vi "Periodic Tasks.vi"(8 "error in":errorcluster) -> (0 "error out":errorcluster)   [LabVIEW 2018]
doc: "This VI runs in parallel to other tasks. It can contain as many user-defined periodic loops as you need. These can carry out PID or other sorts of timed response."
uses:
  <vilib>/Rock Robotics/WPI/Joystick/WPI_JoystickDevRef.ctl
  <vilib>/Rock Robotics/WPI/Joystick/WPI_JoystickDeviceEnum.ctl
  <vilib>/Rock Robotics/WPI/RobotDrive/WPI_RobotDriveDevRef.ctl
  <vilib>/Rock Robotics/WPI/MotorControl/WPI_MotorControlDeviceRef.ctl
  <vilib>/Rock Robotics/WPI/MotorControl/WPI_MotorControlType.ctl
  <vilib>/Rock Robotics/SystemInterfaces/DIO/FPGA_DIOPWMChannel.ctl
  <vilib>/Rock Robotics/WPI/PWM/WPI_PWMDeadband.ctl
  <vilib>/Rock Robotics/SystemInterfaces/DIO/FPGA_DIOChannel.ctl
  <vilib>/Rock Robotics/WPI/Solenoid/WPI_SolenoidDevRef.ctl
  <vilib>/Rock Robotics/WPI/Solenoid/WPI_SolenoidChannel.ctl
  <vilib>/Rock Robotics/WPI/DigitalInput/WPI_DigitalInputDevRef.ctl
  Vision States.ctl
  <vilib>/Rock Robotics/WPI/DriverStation/WPI_DriverStationRobotMode2.ctl
  Hatch Retainer States.ctl
  HAB Bk Spd Motor States.ctl
  Hatch Kicking States.ctl
  <vilib>/Rock Robotics/WPI/Solenoid/WPI_SolenoidValue.ctl
  <vilib>/Rock Robotics/WPI/ThirdParty/Phoenix-LabVIEW/Motor Controller/Controls/CTRE_Phoenix_MotorControl_ControlMode.ctl
  <vilib>/Rock Robotics/WPI/ThirdParty/Phoenix-LabVIEW/Motor Controller/Controls/CTRE_Phoenix_MotorControl_MotionProfileTrajectoryPoint.ctl
  <vilib>/Rock Robotics/WPI/Utilities/WPI_GetSetVariantRefNum.vi
  <vilib>/Rock Robotics/WPI/ThirdParty/Phoenix-LabVIEW/Motor Controller/Get/CTRE_Phoenix_MotorController_GetQuadratureData.vi
  Robot Global Data.vi
  <vilib>/Rock Robotics/Network Tables/NT Write Boolean.vi
  <vilib>/Rock Robotics/WPI/Solenoid/WPI_SolenoidSetEnum.vi
  <vilib>/addons/control/pid/pid.llb/PID (DBL).vi
  <vilib>/Rock Robotics/Network Tables/NT Write Number.vi
  <vilib>/Rock Robotics/WPI/ThirdParty/Phoenix-LabVIEW/Motor Controller/Closed Loop/Motion Profile/CTRE_Phoenix_MotorControl_BufferedTrajectoryPointStream_WriteAll.vi
  <vilib>/Rock Robotics/Network Tables/NT Read Number.vi
  <vilib>/addons/control/pid/NI_PID_pid.lvlib
panel:
  in  "FRDriveMotorDevRef":T1={"DeviceStatus"={"status"=FALSE, "code"=0, "source"=""}, "Type"=enum."PWM", "PWM"={"PWM Channel"=enum."Invalid", "DeadBand"={"Name"="", "maxPositivePwm"=0, "minPositivePwm"=0, "centerPwm"=0, "maxNegativePwm"=0, "minNegativePwm"=0, "angularRange"=0}}, "CAN"={"Device Number"=0, "SetOutput VI Ref"=variant(refnum<vi> refnum), "GetOutput VI Ref"=variant(refnum<vi> refnum), "Enable VI Ref"=variant(refnum<vi> refnum), "Disable VI Ref"=variant(refnum<vi> refnum), "Data"=variant}, "Invert"=FALSE, "DIO PWM"={"PWM \"Enable\" Channel"=enum."Invalid", "DIOChannel"=enum."Invalid", "PWM Rate"=0.0}}
  in  "FLDriveMotorDevRef":T1={"DeviceStatus"={"status"=FALSE, "code"=0, "source"=""}, "Type"=enum."PWM", "PWM"={"PWM Channel"=enum."Invalid", "DeadBand"={"Name"="", "maxPositivePwm"=0, "minPositivePwm"=0, "centerPwm"=0, "maxNegativePwm"=0, "minNegativePwm"=0, "angularRange"=0}}, "CAN"={"Device Number"=0, "SetOutput VI Ref"=variant(refnum<vi> refnum), "GetOutput VI Ref"=variant(refnum<vi> refnum), "Enable VI Ref"=variant(refnum<vi> refnum), "Disable VI Ref"=variant(refnum<vi> refnum), "Data"=variant}, "Invert"=FALSE, "DIO PWM"={"PWM \"Enable\" Channel"=enum."Invalid", "DIOChannel"=enum."Invalid", "PWM Rate"=0.0}}
  in  "HAB3DriveModuleMotorDevRef 2":T1={"DeviceStatus"={"status"=FALSE, "code"=0, "source"=""}, "Type"=enum."PWM", "PWM"={"PWM Channel"=enum."Invalid", "DeadBand"={"Name"="", "maxPositivePwm"=0, "minPositivePwm"=0, "centerPwm"=0, "maxNegativePwm"=0, "minNegativePwm"=0, "angularRange"=0}}, "CAN"={"Device Number"=0, "SetOutput VI Ref"=variant(refnum<vi> refnum), "GetOutput VI Ref"=variant(refnum<vi> refnum), "Enable VI Ref"=variant(refnum<vi> refnum), "Disable VI Ref"=variant(refnum<vi> refnum), "Data"=variant}, "Invert"=FALSE, "DIO PWM"={"PWM \"Enable\" Channel"=enum."Invalid", "DIOChannel"=enum."Invalid", "PWM Rate"=0.0}}
  in  "BkSpdAdjusterMotorDevRef":T1={"DeviceStatus"={"status"=FALSE, "code"=0, "source"=""}, "Type"=enum."PWM", "PWM"={"PWM Channel"=enum."Invalid", "DeadBand"={"Name"="", "maxPositivePwm"=0, "minPositivePwm"=0, "centerPwm"=0, "maxNegativePwm"=0, "minNegativePwm"=0, "angularRange"=0}}, "CAN"={"Device Number"=0, "SetOutput VI Ref"=variant(refnum<vi> refnum), "GetOutput VI Ref"=variant(refnum<vi> refnum), "Enable VI Ref"=variant(refnum<vi> refnum), "Disable VI Ref"=variant(refnum<vi> refnum), "Data"=variant}, "Invert"=FALSE, "DIO PWM"={"PWM \"Enable\" Channel"=enum."Invalid", "DIOChannel"=enum."Invalid", "PWM Rate"=0.0}}
  in  "HABAssisterSolenoidDevRef":T6={"DevStatus"={"status"=FALSE, "code"=0, "source"=""}, "Pneumatics Control Module"=0, "Forward Solenoid Channel"=enum."Invalid", "Reverse Solenoid Channel"=enum."Invalid"}
  out "Right Traj. Pts Array":dbl[][](array[numeric])
  out "Left Traj. Pts Array":dbl[][](array[numeric])
  in  "Back HAB 3 Limit Switch":T8={"DevStatus"={"status"=FALSE, "code"=0, "source"=""}, "DIO Channel"=enum."Invalid"}
  in  "Front HAB 3 Limit Switch":T8={"DevStatus"={"status"=FALSE, "code"=0, "source"=""}, "DIO Channel"=enum."Invalid"}
  in  "BottomRetainerSwitchDevRef":T8={"DevStatus"={"status"=FALSE, "code"=0, "source"=""}, "DIO Channel"=enum."Invalid"}
  in  "TopRetainerSwitchDevRef":T8={"DevStatus"={"status"=FALSE, "code"=0, "source"=""}, "DIO Channel"=enum."Invalid"}
  in  "HatchRetainerMotorDevRef":T1={"DeviceStatus"={"status"=FALSE, "code"=0, "source"=""}, "Type"=enum."PWM", "PWM"={"PWM Channel"=enum."Invalid", "DeadBand"={"Name"="", "maxPositivePwm"=0, "minPositivePwm"=0, "centerPwm"=0, "maxNegativePwm"=0, "minNegativePwm"=0, "angularRange"=0}}, "CAN"={"Device Number"=0, "SetOutput VI Ref"=variant(refnum<vi> refnum), "GetOutput VI Ref"=variant(refnum<vi> refnum), "Enable VI Ref"=variant(refnum<vi> refnum), "Disable VI Ref"=variant(refnum<vi> refnum), "Data"=variant}, "Invert"=FALSE, "DIO PWM"={"PWM \"Enable\" Channel"=enum."Invalid", "DIOChannel"=enum."Invalid", "PWM Rate"=0.0}}
  in  "HAB3BackSolenoidDevRef":T6={"DevStatus"={"status"=FALSE, "code"=0, "source"=""}, "Pneumatics Control Module"=0, "Forward Solenoid Channel"=enum."Invalid", "Reverse Solenoid Channel"=enum."Invalid"}
  in  "HAB3FrontSolenoidDevRef":T6={"DevStatus"={"status"=FALSE, "code"=0, "source"=""}, "Pneumatics Control Module"=0, "Forward Solenoid Channel"=enum."Invalid", "Reverse Solenoid Channel"=enum."Invalid"}
  in  "AuxJoystickDevRef":T9={"Device"=enum."USB 1"}
  in  "DriveJoystickDevRef":T9={"Device"=enum."USB 1"}
  in  "HAB3DriveModuleMotorDevRef":T1={"DeviceStatus"={"status"=FALSE, "code"=0, "source"=""}, "Type"=enum."PWM", "PWM"={"PWM Channel"=enum."Invalid", "DeadBand"={"Name"="", "maxPositivePwm"=0, "minPositivePwm"=0, "centerPwm"=0, "maxNegativePwm"=0, "minNegativePwm"=0, "angularRange"=0}}, "CAN"={"Device Number"=0, "SetOutput VI Ref"=variant(refnum<vi> refnum), "GetOutput VI Ref"=variant(refnum<vi> refnum), "Enable VI Ref"=variant(refnum<vi> refnum), "Disable VI Ref"=variant(refnum<vi> refnum), "Data"=variant}, "Invert"=FALSE, "DIO PWM"={"PWM \"Enable\" Channel"=enum."Invalid", "DIOChannel"=enum."Invalid", "PWM Rate"=0.0}}
  in  "LifterSolenoidDevRef":T6={"DevStatus"={"status"=FALSE, "code"=0, "source"=""}, "Pneumatics Control Module"=0, "Forward Solenoid Channel"=enum."Invalid", "Reverse Solenoid Channel"=enum."Invalid"}
  in  "DriveJoystickDevRef":T9={"Device"=enum."USB 1"}
  in  "HatchCollectorMotorDevRef":T1={"DeviceStatus"={"status"=FALSE, "code"=0, "source"=""}, "Type"=enum."PWM", "PWM"={"PWM Channel"=enum."Invalid", "DeadBand"={"Name"="", "maxPositivePwm"=0, "minPositivePwm"=0, "centerPwm"=0, "maxNegativePwm"=0, "minNegativePwm"=0, "angularRange"=0}}, "CAN"={"Device Number"=0, "SetOutput VI Ref"=variant(refnum<vi> refnum), "GetOutput VI Ref"=variant(refnum<vi> refnum), "Enable VI Ref"=variant(refnum<vi> refnum), "Disable VI Ref"=variant(refnum<vi> refnum), "Data"=variant}, "Invert"=FALSE, "DIO PWM"={"PWM \"Enable\" Channel"=enum."Invalid", "DIOChannel"=enum."Invalid", "PWM Rate"=0.0}}
  in  "AuxJoystickDevRef":T9
  in  "RetainerSolenoidDevRef":T6={"DevStatus"={"status"=FALSE, "code"=0, "source"=""}, "Pneumatics Control Module"=0, "Forward Solenoid Channel"=enum."Invalid", "Reverse Solenoid Channel"=enum."Invalid"}
  in  "KickerSolenoidDevRef":T6={"DevStatus"={"status"=FALSE, "code"=0, "source"=""}, "Pneumatics Control Module"=0, "Forward Solenoid Channel"=enum."Invalid", "Reverse Solenoid Channel"=enum."Invalid"}
  in  "Drive Motors":T11={"DevStatus"={"status"=FALSE, "code"=0, "source"=""}, "Motors[]"=[], "Square Inputs"=FALSE, "Max Output"=1.0}
  in  "AuxJoystickDevRef":T9={"Device"=enum."USB 1"}
  in  "DriveJoystickDevRef":T9
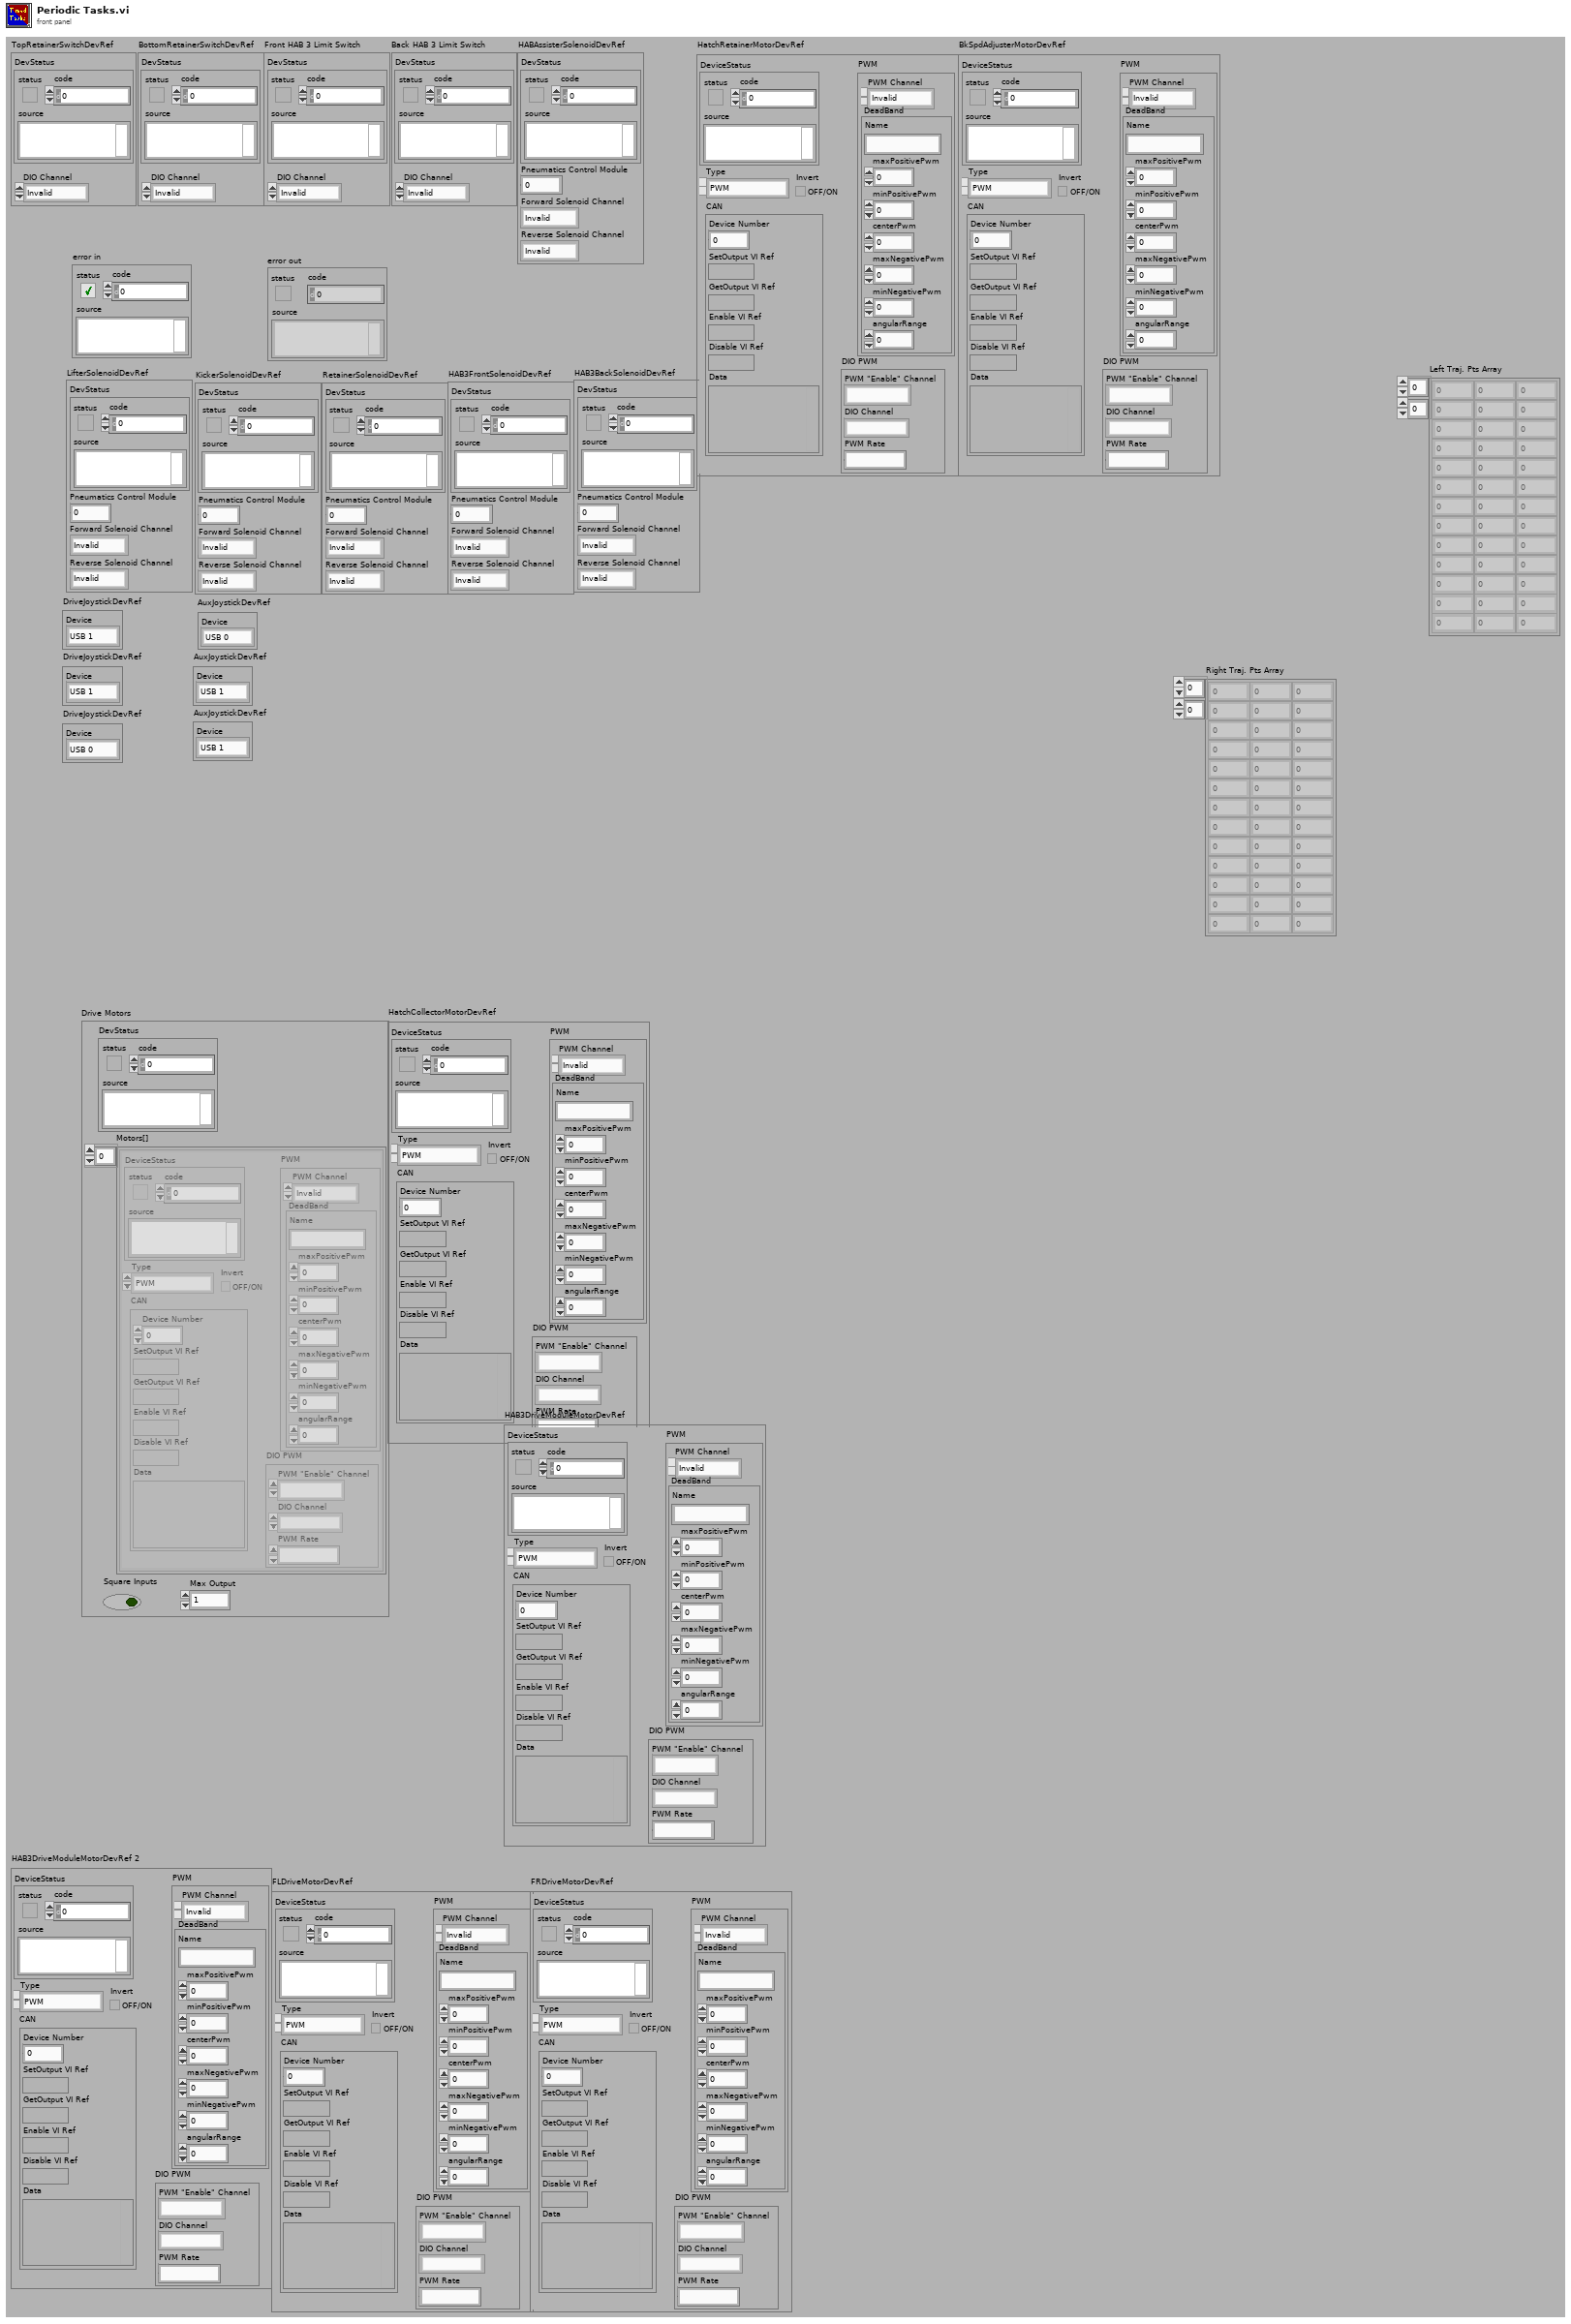
[diagram p1: front panel]
types:
  T1 = typedef "WPI_MotorControlDeviceRef.ctl" = cluster{"DeviceStatus":errorcluster, "Type":T2, "PWM":cluster{"PWM Channel":T3, "DeadBand":T4}, "CAN":cluster{"Device Number":u8, "SetOutput VI Ref":variant, "GetOutput VI Ref":variant, "Enable VI Ref":variant, "Disable VI Ref":variant, "Data":variant}, "Invert":bool, "DIO PWM":cluster{"PWM \"Enable\" Channel":T3, "DIOChannel":T5, "PWM Rate":dbl}}
  T2 = typedef "WPI_MotorControlType.ctl" = enum16{"PWM", "CAN", "DIO PWM"}
  T3 = typedef "FPGA_DIOPWMChannel.ctl" = enum8{"PWM 0", "PWM 1", "PWM 2", "PWM 3", "PWM 4", "PWM 5", "PWM 6", "PWM 7", "PWM 8", "PWM 9", "PWM MXP 0", "PWM MXP 1", "PWM MXP 2", "PWM MXP 3", "PWM MXP 4", "PWM MXP 5", "PWM MXP 6", "PWM MXP 7", "PWM MXP 8", "PWM MXP 9", "Invalid"}
  T4 = typedef "WPI_PWMDeadband.ctl" = cluster{"Name":string, "maxPositivePwm":i32, "minPositivePwm":i32, "centerPwm":i32, "maxNegativePwm":i32, "minNegativePwm":i32, "angularRange":u16}
  T5 = typedef "FPGA_DIOChannel.ctl" = enum8{"DIO 0", "DIO 1", "DIO 2", "DIO 3", "DIO 4", "DIO 5", "DIO 6", "DIO 7", "DIO 8", "DIO 9", "DIO MXP 0", "DIO MXP 1", "DIO MXP 2", "DIO MXP 3", "DIO MXP 4", "DIO MXP 5", "DIO MXP 6", "DIO MXP 7", "DIO MXP 8", "DIO MXP 9", "DIO MXP 10", "DIO MXP 11", "DIO MXP 12", "DIO MXP 13", "DIO MXP 14", "DIO MXP 15", "SPI Port CS1", "SPI Port CS2", "SPI Port CS3", "SPI Port MISO", "SPI Port MOSI", "Invalid"}
  T6 = typedef "WPI_SolenoidDevRef.ctl" = cluster{"DevStatus":errorcluster, "Pneumatics Control Module":u8, "Forward Solenoid Channel":T7, "Reverse Solenoid Channel":T7}
  T7 = typedef "WPI_SolenoidChannel.ctl" = enum8{"Solenoid 0", "Solenoid 1", "Solenoid 2", "Solenoid 3", "Solenoid 4", "Solenoid 5", "Solenoid 6", "Solenoid 7", "Invalid"}
  T8 = typedef "WPI_DigitalInputDevRef.ctl" = cluster{"DevStatus":errorcluster, "DIO Channel":T5}
  T9 = typedef "WPI_JoystickDevRef.ctl" = cluster{"Device":T10}
  T10 = typedef "WPI_JoystickDeviceEnum.ctl" = enum16{"USB 0", "USB 1", "USB 2", "USB 3", "USB 4", "USB 5"}
  T11 = typedef "WPI_RobotDriveDevRef.ctl" = cluster{"DevStatus":errorcluster, "Motors[]":T1[], "Square Inputs":bool, "Max Output":dbl}
  T12 = typedef "Hatch Kicking States.ctl" = enum16{"Ready", "Stop Retaining Hatch", "Kick Hatch"}
  T13 = typedef "HAB Bk Spd Motor States.ctl" = enum16{"Fully Up", "Going Down", "Fully Down", "Going Up"}
  T14 = typedef "Hatch Retainer States.ctl" = enum16{"Fully Down (not retained)", "Going Up", "Fully Up (retained)", "Going Down"}
  T15 = cluster{"X Button":i32, "A Button":i32, "B Button":i32, "Y Button":i32, "LB Button":i32, "RB Button":i32, "LT Button":i32, "RT Button":i32, "BACK Button":i32, "START Button":i32, "LJ Click Button":i32, "RJ Click Button":i32}
  T16 = cluster{"Left X":i32, "Left Y":i32, "Right X":i32, "Right Y":i32}
  T17 = typedef "WPI_DriverStationRobotMode2.ctl" = enum16{"Autonomous Disabled", "Autonomous Enabled", "Teleop Disabled", "Teleop Enabled", "Disconnected", "Finish", "Test Disabled", "Test Enabled", "Emergency Stopped"}
  T18 = cluster{"offsetAngle H":dbl, "offsetAngle V":dbl, "area":dbl, "skew":dbl, "shortest side (pxls)":dbl, "longest side (pxls)":dbl}
  T19 = typedef "Vision States.ctl" = enum16{"Ready", "Forward Until Target at Edge", "Vision Track"}
  T20 = cluster{"A Button":i32, "B Button":i32, "X Button":i32, "Y Button":i32, "LB Button":i32, "RB Button":i32, "BACK Button":i32, "START Button":i32, "LJ Click Button":i32, "RJ Click Button":i32}
  T21 = cluster{"Left X":i32, "Left Y":i32, "Right X":i32, "Right Y":i32, "RT Button":i32, "LT Button":i32}
  T22 = cluster{"MotorControlDevRef":T1, "MotorControlDevRef":T1}
  T23 = typedef "WPI_GyroDevRef.ctl" = cluster{"DevStatus":errorcluster, "Analog Channel":T24, "Gain (VoltsPerDegree/Second)":dbl, "Gyro Type":enum16{"Analog", "XRS450"}, "Handle":i32, "SPI Bus":T25, "Device Found":bool, "Sample Rate":dbl, "Calibrate On Open":bool, "Offset":dbl}
  T24 = typedef "FPGA_AIChannel.ctl" = enum8{"AI 0", "AI 1", "AI 2", "AI 3", "AI MXP 0", "AI MXP 1", "AI MXP 2", "AI MXP 3", "Invalid"}
  T25 = typedef "spi_bus.ctl" = enum16{"SPI On-Board, CS0", "SPI On-Board, CS1", "SPI On-Board, CS2", "SPI On-Board, CS3", "SPI MXP", "Invalid"}
  T26 = cluster{"Front Drive Motors":cluster{"FLDriveMotor":T1, "FRDriveMotor":T1}, "HAB3DriveModuleMotorDevRef 2":T1, "DriveJoystickDevRef":T9, "AuxJoystickDevRef":T9, "Drive Axes":dbl[], "Drive Buttons":bool[], "Drive POVs":i16[], "Aux Axes":dbl[], "Aux Buttons":bool[], "Aux POVs":i16[], "Robot Mode":T17, "Drive Motors":T11, "Drive Axes Indexes":cluster{"Left X":i32, "Left Y":i32, "Right X":i32, "Right Y":i32, "RT Button":i32, "LT Button":i32}, "Drive Button Indexes":cluster{"A Button":i32, "B Button":i32, "X Button":i32, "Y Button":i32, "LB Button":i32, "RB Button":i32, "BACK Button":i32, "START Button":i32, "LJ Click Button":i32, "RJ Click Button":i32}, "Joystick VS Vision Latch":bool, "Vision States":T19, "limelight":cluster{"offsetAngle H":dbl, "offsetAngle V":dbl, "area":dbl, "skew":dbl, "shortest side (pxls)":dbl, "longest side (pxls)":dbl}, "Vision Track Mode Override":bool, "T = Motion Profile, F = Percent Output":bool, "Arcade Drive?":bool, "Start Motion Profile?":bool}
  T27 = cluster{"TopRetainerSwitchDevRef":T8, "BottomRetainerSwitchDevRef":T8, "HatchRetainerMotorDevRef":T1, "LifterSolenoidDevRef":T6, "DriveJoystickDevRef":T9, "KickerSolenoidDevRef":T6, "RetainerSolenoidDevRef":T6, "AuxJoystickDevRef":T9, "HatchCollectorMotorDevRef":T1, "Drive Axes":dbl[], "Drive Buttons":bool[], "Drive POVs":i16[], "Aux Axes":dbl[], "Aux Buttons":bool[], "Aux POVs":i16[], "Robot Mode":T17, "Aux Joystick Indexes":cluster{"Left X":i32, "Left Y":i32, "Right X":i32, "Right Y":i32}, "Aux Button Indexes":cluster{"X Button":i32, "A Button":i32, "B Button":i32, "Y Button":i32, "LB Button":i32, "RB Button":i32, "LT Button":i32, "RT Button":i32, "BACK Button":i32, "START Button":i32, "LJ Click Button":i32, "RJ Click Button":i32}, "Hatch Retainer Move Up/Down":bool, "Hatch Collector Actual Angle":dbl, "Hatch Collector Wanted Angle":dbl, "Hatch Retainer States":T14, "Hatch Kicking States":T12}
  T28 = cluster{"BkSpdAdjusterMotorDevRef":T1, "HABAssisterSolenoidDevRef":T6, "Back HAB 3 Limit Switch":T8, "Front HAB 3 Limit Switch":T8, "HAB3DriveModuleMotorDevRef":T1, "DriveJoystickDevRef":T9, "AuxJoystickDevRef":T9, "HAB3FrontSolenoidDevRef":T6, "HAB3BackSolenoidDevRef":T6, "Drive Axes":dbl[], "Drive Buttons":bool[], "Drive POVs":i16[], "Aux Axes":dbl[], "Aux Buttons":bool[], "Aux POVs":i16[], "Robot Mode":T17, "Aux Joystick Indexes":cluster{"Left X":i32, "Left Y":i32, "Right X":i32, "Right Y":i32}, "Aux Button Indexes":cluster{"X Button":i32, "A Button":i32, "B Button":i32, "Y Button":i32, "LB Button":i32, "RB Button":i32, "LT Button":i32, "RT Button":i32, "BACK Button":i32, "START Button":i32, "LJ Click Button":i32, "RJ Click Button":i32}, "Front Cylinders Latch":bool, "Back Cylinders Latch":bool, "Yaw":dbl, "Pitch":dbl, "Roll":dbl, "HAB Bk Spd Motor States":T13}
  T29 = typedef "CTRE_Phoenix_MotorControl_MotionProfileTrajectoryPoint.ctl" = cluster{"Position":dbl, "Velocity":dbl, "Arbitrary Feed Forward":dbl, "Auxiliary Position":dbl, "Auxiliary Velocity":dbl, "Auxiliary Arbitrary Feed Forward":dbl, "Profile Slot Select":i32, "Auxiliary Profile Slot Select":i32, "isLastPoint?":bool, "Zero Position?":bool, "durationMs":u32, "Use Aux PID?":bool}
  T30 = typedef "Which Robot Enum.ctl" = enum16{"Competition Bot", "Practice Bot", "Code Bot"}
  T31 = typedef "CTRE_Phoenix_MotorControl_BufferedTrajectoryPointStream_DeviceRef.ctl" = cluster{"Handle":u64, "Library Path":path}
  T32 = typedef "WPI_SolenoidValue.ctl" = enum16{"Off", "On", "Forward", "Reverse"}
  T33 = cluster{"proportional gain (Kc)":dbl, "integral time (Ti, min)":dbl, "derivative time (Td, min)":dbl}
  T34 = typedef "CTRE_Phoenix_MotorControl_ControlMode.ctl" = u16
  T35 = cluster{"Yaw":dbl, "Roll":dbl, "Pitch":dbl, "Heading":dbl, "Fused Heading":dbl}
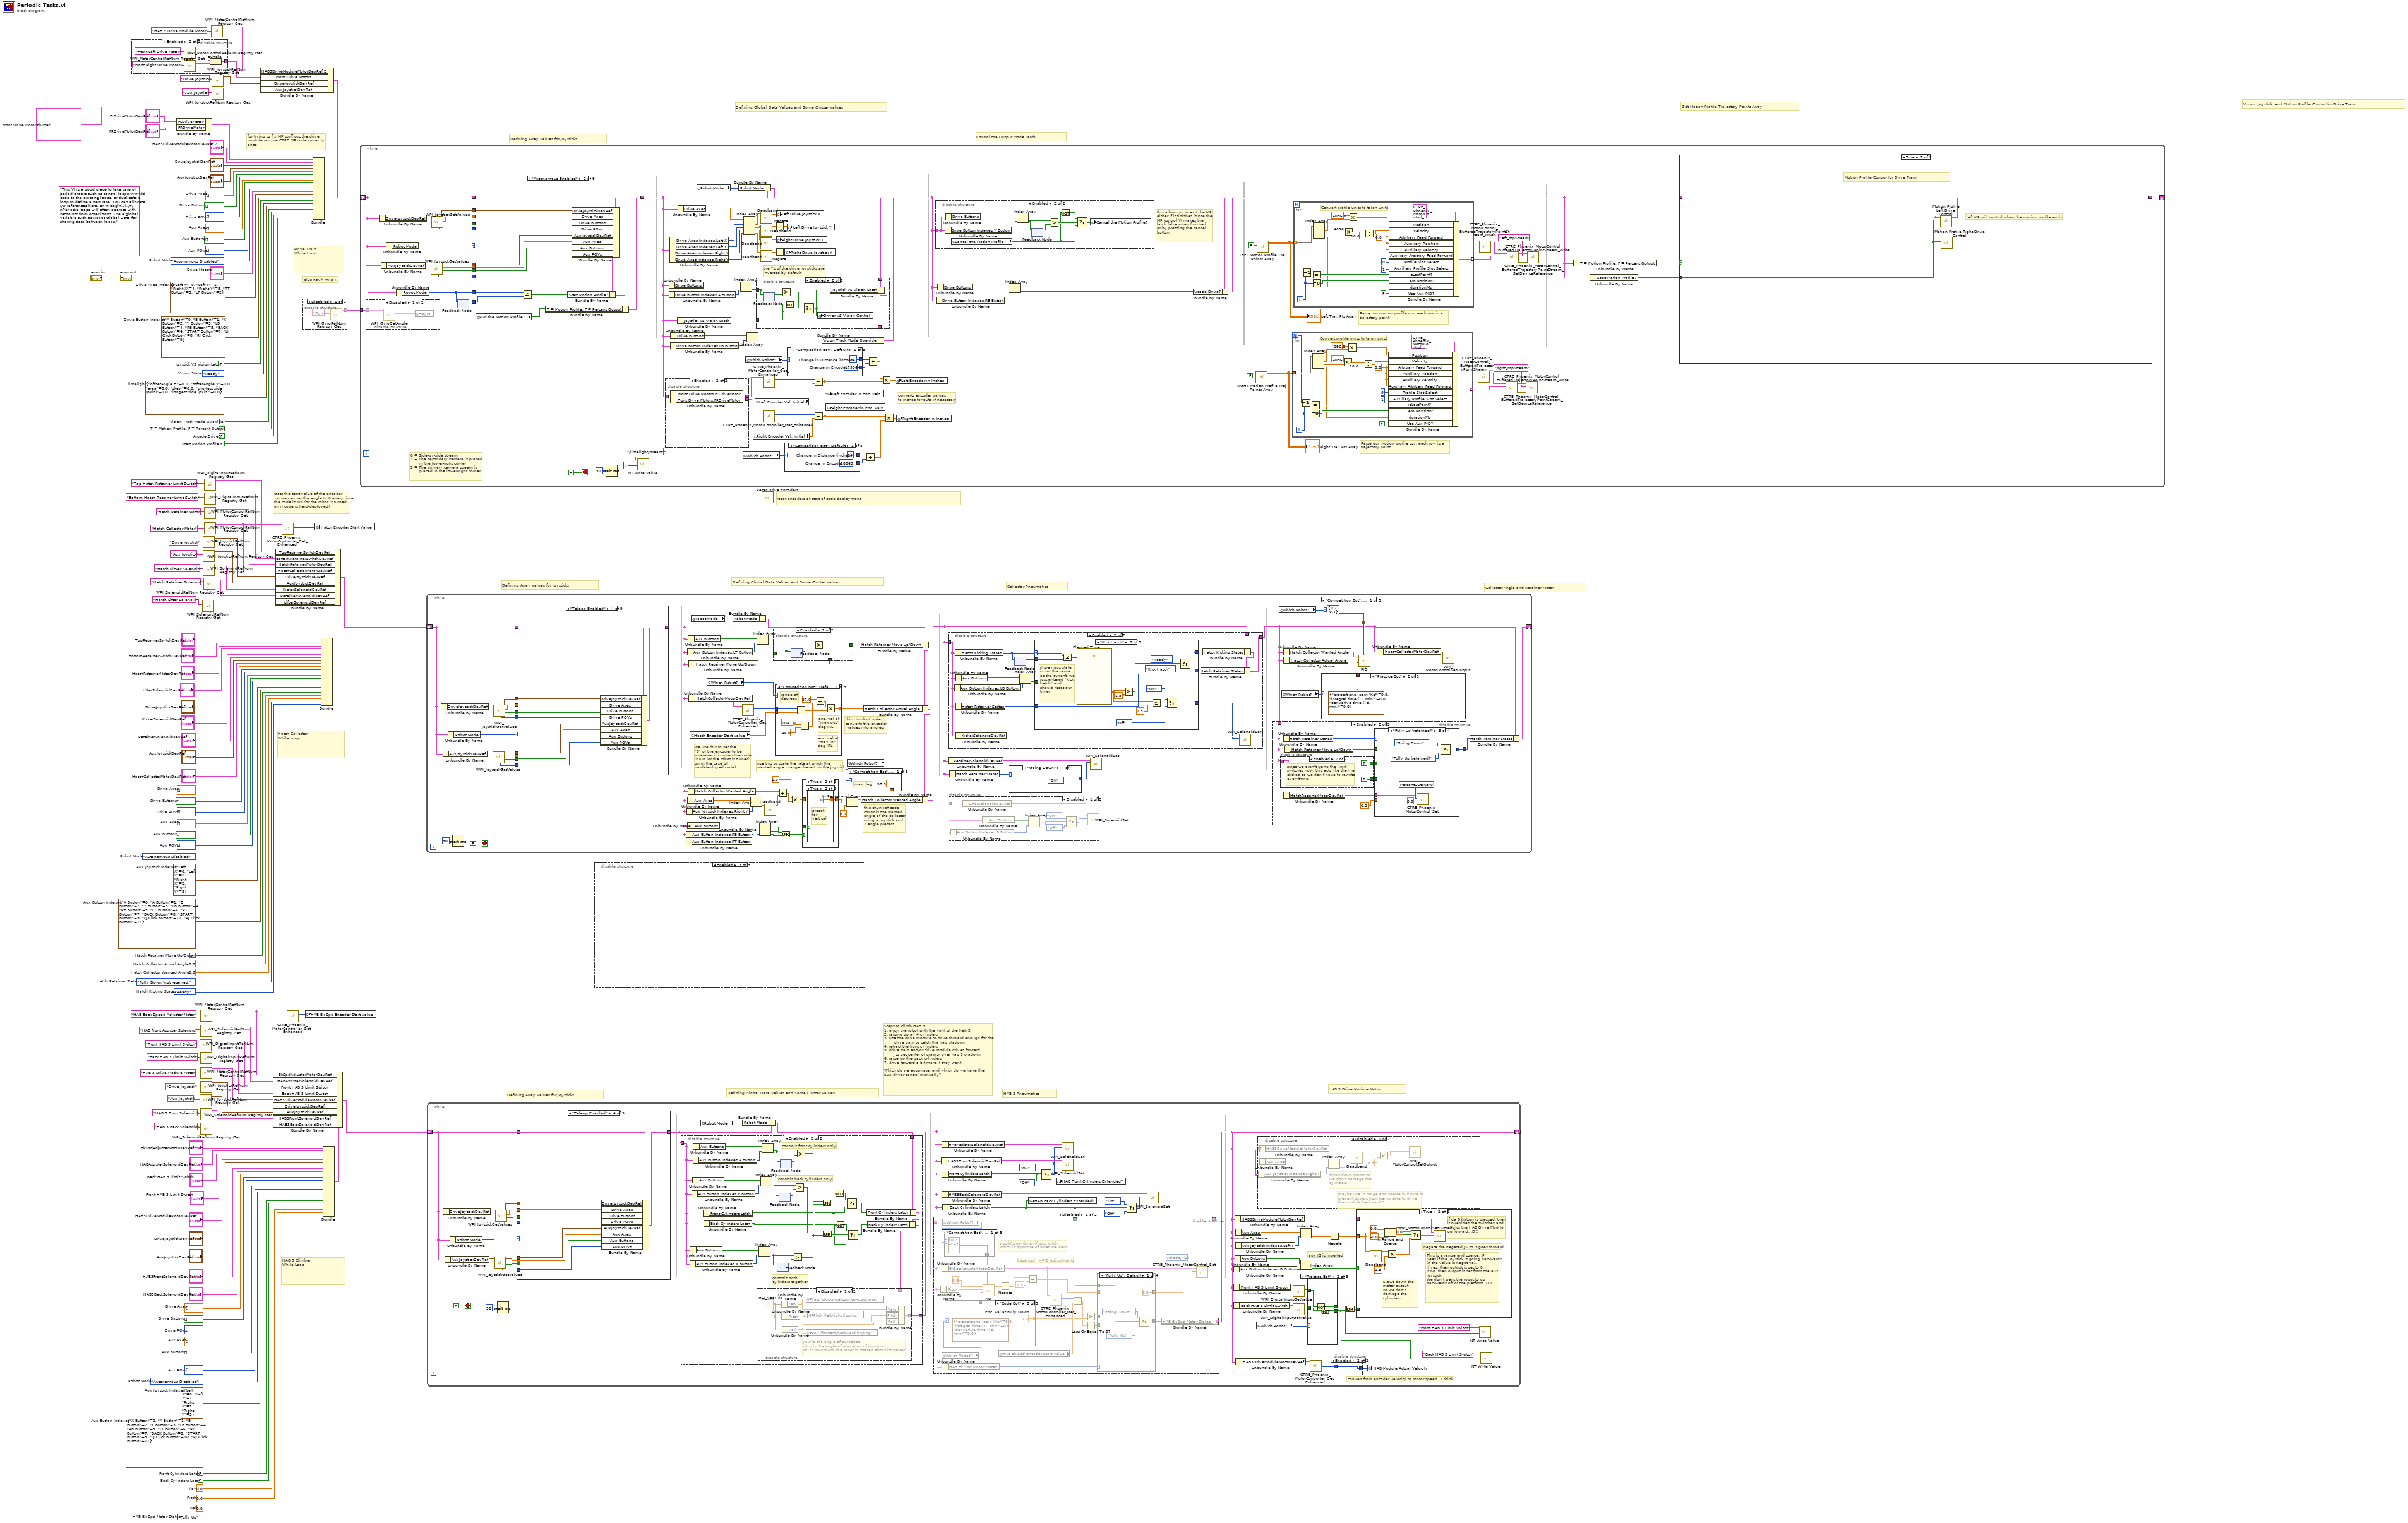
[diagram p0: block diagram]
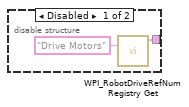
[diagram p2: hidden frame]
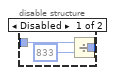
[diagram p3: hidden frame]
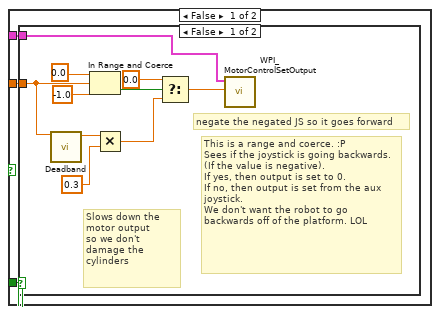
[diagram p4: hidden frame]
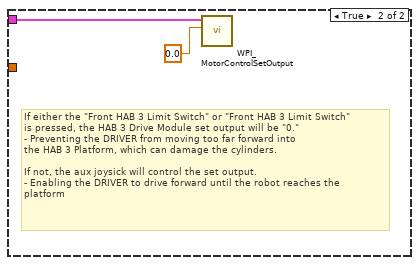
[diagram p5: hidden frame]
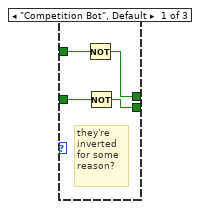
[diagram p6: hidden frame]
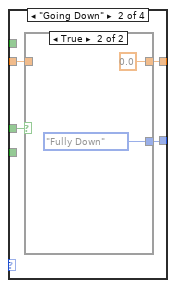
[diagram p8: hidden frame]
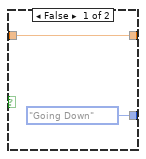
[diagram p9: hidden frame]
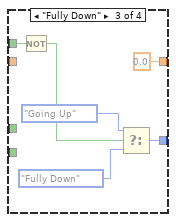
[diagram p10: hidden frame]
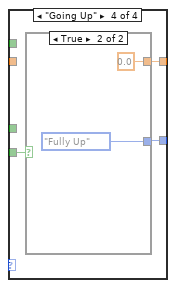
[diagram p11: hidden frame]
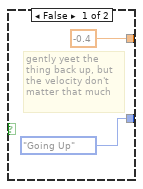
[diagram p12: hidden frame]
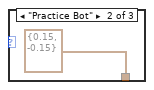
[diagram p13: hidden frame]
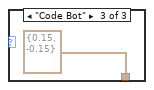
[diagram p14: hidden frame]
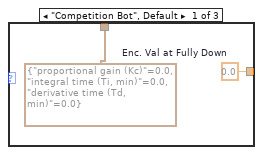
[diagram p15: hidden frame]
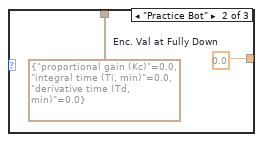
[diagram p16: hidden frame]
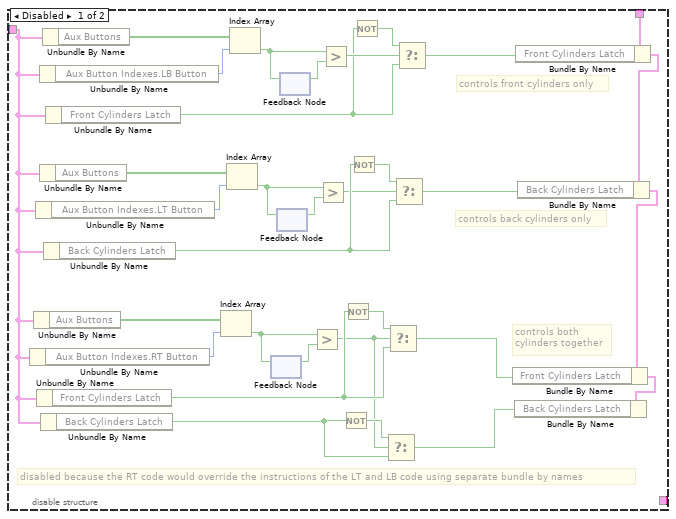
[diagram p18: hidden frame]
diagram:
  w1 = cluster{"FLDriveMotor":T1, "FRDriveMotor":T1} {"FLDriveMotor"={"DeviceStatus"={"status"=FALSE, "code"=0, "source"=""}, "Type"=enum."PWM", "PWM"={"PWM Channel"=enum."Invalid", "DeadBand"={"Name"="", "maxPositivePwm"=0, "minPositivePwm"=0, "centerPwm"=0, "maxNegativePwm"=0, "minNegativePwm"=0, "angularRange"=0}}, "CAN"={"Device Number"=0, "SetOutput VI Ref"=variant(refnum<vi> refnum), "GetOutput VI Ref"=variant(refnum<vi> refnum), "Enable VI Ref"=variant(refnum<vi> refnum), "Disable VI Ref"=variant(refnum<vi> refnum), "Data"=variant}, "Invert"=FALSE, "DIO PWM"={"PWM \"Enable\" Channel"=enum."Invalid", "DIOChannel"=enum."Invalid", "PWM Rate"=0.0}}, "FRDriveMotor"={"DeviceStatus"={"status"=FALSE, "code"=0, "source"=""}, "Type"=enum."PWM", "PWM"={"PWM Channel"=enum."Invalid", "DeadBand"={"Name"="", "maxPositivePwm"=0, "minPositivePwm"=0, "centerPwm"=0, "maxNegativePwm"=0, "minNegativePwm"=0, "angularRange"=0}}, "CAN"={"Device Number"=0, "SetOutput VI Ref"=variant(refnum<vi> refnum), "GetOutput VI Ref"=variant(refnum<vi> refnum), "Enable VI Ref"=variant(refnum<vi> refnum), "Disable VI Ref"=variant(refnum<vi> refnum), "Data"=variant}, "Invert"=FALSE, "DIO PWM"={"PWM \"Enable\" Channel"=enum."Invalid", "DIOChannel"=enum."Invalid", "PWM Rate"=0.0}}}  # Front Drive Motors
  w9 = FALSE  # Start Motion Profile?
  w10 = FALSE  # Arcade Drive?
  w11 = Hatch_Kicking_States."Ready"  # Hatch Kicking States
  w12 = HAB_Bk_Spd_Motor_States."Fully Up"  # HAB Bk Spd Motor States
  w17 = 0.0  # Roll
  w18 = 0.0  # Pitch
  w19 = 0.0  # Yaw
  w29 = Hatch_Retainer_States."Fully Down (not retained)"  # Hatch Retainer States
  w39 = FALSE  # T = Motion Profile, F = Percent Output
  w41 = 0.0  # Hatch Collector Wanted Angle
  w42 = FALSE  # Back Cylinders Latch
  w43 = FALSE  # Front Cylinders Latch
  w44 = T15 {"X Button"=0, "A Button"=1, "B Button"=2, "Y Button"=3, "LB Button"=4, "RB Button"=5, "LT Button"=6, "RT Button"=7, "BACK Button"=8, "START Button"=9, "LJ Click Button"=10, "RJ Click Button"=11}  # Aux Button Indexes
  w45 = T16 {"Left X"=0, "Left Y"=1, "Right X"=2, "Right Y"=3}  # Aux Joystick Indexes
  w46 = WPI_DriverStationRobotMode2."Autonomous Disabled"  # Robot Mode
  w47 = i16[] []  # Aux POVs
  w48 = bool[] []  # Aux Buttons
  w49 = dbl[] []  # Aux Axes
  w50 = i16[] []  # Drive POVs
  w51 = bool[] []  # Drive Buttons
  w52 = dbl[] []  # Drive Axes
  w75 = 0.0  # Hatch Collector Actual Angle
  w76 = FALSE  # Hatch Retainer Move Up/Down
  w77 = T15 {"X Button"=0, "A Button"=1, "B Button"=2, "Y Button"=3, "LB Button"=4, "RB Button"=5, "LT Button"=6, "RT Button"=7, "BACK Button"=8, "START Button"=9, "LJ Click Button"=10, "RJ Click Button"=11}  # Aux Button Indexes
  w78 = T16 {"Left X"=0, "Left Y"=1, "Right X"=2, "Right Y"=3}  # Aux Joystick Indexes
  w82 = WPI_DriverStationRobotMode2."Autonomous Disabled"  # Robot Mode
  w83 = i16[] []  # Aux POVs
  w84 = bool[] []  # Aux Buttons
  w85 = dbl[] []  # Aux Axes
  w86 = i16[] []  # Drive POVs
  w87 = bool[] []  # Drive Buttons
  w88 = dbl[] []  # Drive Axes
  w102 = FALSE  # Vision Track Mode Override
  w103 = T18 {"offsetAngle H"=0.0, "offsetAngle V"=0.0, "area"=0.0, "skew"=0.0, "shortest side (pxls)"=0.0, "longest side (pxls)"=0.0}  # limelight
  w104 = Vision_States."Ready"  # Vision States
  w105 = FALSE  # Joystick VS Vision Latch
  w106 = T20 {"A Button"=0, "B Button"=1, "X Button"=2, "Y Button"=3, "LB Button"=4, "RB Button"=5, "BACK Button"=6, "START Button"=7, "LJ Click Button"=8, "RJ Click Button"=9}  # Drive Button Indexes
  w108 = T21 {"Left X"=0, "Left Y"=1, "Right X"=4, "Right Y"=5, "RT Button"=3, "LT Button"=2}  # Drive Axes Indexes
  w112 = i16[] []  # Aux POVs
  w113 = bool[] []  # Aux Buttons
  w114 = dbl[] []  # Aux Axes
  w111 = WPI_DriverStationRobotMode2."Autonomous Disabled"  # Robot Mode
  w115 = i16[] []  # Drive POVs
  w116 = bool[] []  # Drive Buttons
  w117 = dbl[] []  # Drive Axes
  (unwired) "This VI is a good place to take care of periodic tasks such as control loops.\n\nAdd code to the existing loops, or duplicate a loop to define a new rate. You can allocate I/O references here, or in Begin.vi.\n\nPeriodic loops will often operate with setpoints from other loops. Use a global variable such as Robot Global Data for sharing data between loops."
  # "HAB 3 Drive Module Motor"
  # "HAB 3 Pneumatics"
  # "Steps to climb HAB 3\n1. align the robot with the front of the hab 3\n2. raising up all 4 cylinders\n3. use the drive module to drive forward enough for the \n        drive train to catch the hab platform\n4. retract the front cylinders\n5. drive train and/or drive module drives forward \n         to get center of gravity over hab 3 platform\n6. raise up the back cylinders\n7. drive forward a bit more if they want\n\nWhich do we automate, and which do we have the \naux driver control manually?"
  # "Defining Global Data Values and Some Cluster Values"
  # "Defining Array Values for Joysticks"
  # "Collector Angle and Retainer Motor"
  # "Collector Pneumatics"
  # "Defining Global Data Values and Some Cluster Values"
  # "Defining Array Values for Joysticks"
  # "for trying to fix MP stuff cuz the drive\nmodule ran the CTRE MP code correctly\nonce"
  # "reset encoders at start of code deployment"
  # "Get Motion Profile Trajectory Points Array"
  # "Control the Output Mode Latch"
  # "plus navX mxp :-)"
  # "Gets the start value of the encoder\n so we can set the angle to 0 every time\nthe code is run (or the robot is turned\non if code is hard-deployed)"
  # "HAB 3 Climber\nWhile Loop"
  # "Hatch Collector\nWhile Loop"
  # "Drive Train\nWhile Loop"
  # "Vision, Joystick, and Motion Profile Control for Drive Train"
  # "Defining Array Values for Joysticks"
  # "Defining Global Data Values and Some Cluster Values"
  n1 = disable-structure shown="Enabled" {
    disable-tunnel: [w126 w129] -> w109
    frame Disabled {
      n2 = call <vilib>:"WPI_RobotDriveRefNum Registry Get.vi"("refnum name"="Drive Motors") -> ("RobotDriveDevRef"=w126:T11)  [unwired: 9 in, 1 out]
    }
    frame Enabled {
      n3 = call <vilib>:"WPI_MotorControlRefNum Registry Get.vi"("refnum name"="Front Left Drive Motor") -> ("MotorControlDevRef"=w130:T1)  [unwired: 9 in, 1 out]
      n4 = call <vilib>:"WPI_MotorControlRefNum Registry Get.vi"("refnum name"="Front Right Drive Motor") -> ("MotorControlDevRef"=w131:T1)  [unwired: 9 in, 1 out]
      n5 = Bundle("MotorControlDevRef"=w130, "MotorControlDevRef"=w131) -> (w129:T22)  [unwired: 1 in]
    }
  }
  n6 = Bundle By Name(cluster=w1, "FLDriveMotor"="FLDriveMotorDevRef", "FRDriveMotor"="FRDriveMotorDevRef") -> (w2:cluster{"FLDriveMotor":T1, "FRDriveMotor":T1})
  n7 = call <vilib>:"WPI_DigitalInputRefNum Registry Get.vi"("refnum name"="Front HAB 3 Limit Switch") -> ("DigitalInputDevRef"=w24:T8)  [unwired: 9 in, 1 out]
  n8 = call <vilib>:"WPI_JoystickRefNum Registry Get.vi"("refnum name"="Aux Joystick") -> ("JoystickDevRef"=w56:T9)  [unwired: 9 in, 1 out]
  n9 = call <vilib>:"WPI_SolenoidRefNum Registry Get.vi"("refnum name"="HAB Front Assister Solenoid") -> ("SolenoidDevRef"=w20:T6)  [unwired: 9 in, 1 out]
  n10 = call <vilib>:"WPI_DigitalInputRefNum Registry Get.vi"("refnum name"="Back HAB 3 Limit Switch") -> ("DigitalInputDevRef"=w23:T8)  [unwired: 9 in, 1 out]
  n11 = call <vilib>:"WPI_MotorControlRefNum Registry Get.vi"("refnum name"="HAB 3 Drive Module Motor") -> ("MotorControlDevRef"=w54:T1)  [unwired: 9 in, 1 out]
  n12 = call <vilib>:"WPI_JoystickRefNum Registry Get.vi"("refnum name"="Drive Joystick") -> ("JoystickDevRef"=w55:T9)  [unwired: 9 in, 1 out]
  n13 = call <vilib>:"WPI_SolenoidRefNum Registry Get.vi"("refnum name"="HAB 3 Front Solenoid") -> ("SolenoidDevRef"=w57:T6)  [unwired: 9 in, 1 out]
  n14 = call <vilib>:"WPI_MotorControlRefNum Registry Get.vi"("refnum name"="HAB Back Speed Adjuster Motor") -> ("MotorControlDevRef"=w13:T1)  [unwired: 9 in, 1 out]
  n15 = call <vilib>:"WPI_SolenoidRefNum Registry Get.vi"("refnum name"="HAB 3 Back Solenoid") -> ("SolenoidDevRef"=w58:T6)  [unwired: 9 in, 1 out]
  n16 = call <vilib>:"WPI_SolenoidRefNum Registry Get.vi"("refnum name"="Hatch Lifter Solenoid") -> ("SolenoidDevRef"=w71:T6)  [unwired: 9 in, 1 out]
  n17 = call <vilib>:"WPI_JoystickRefNum Registry Get.vi"("refnum name"="Aux Joystick") -> ("JoystickDevRef"=w93:T9)  [unwired: 9 in, 1 out]
  n18 = call <vilib>:"WPI_JoystickRefNum Registry Get.vi"("refnum name"="Drive Joystick") -> ("JoystickDevRef"=w79:T9)  [unwired: 9 in, 1 out]
  n19 = call <vilib>:"WPI_SolenoidRefNum Registry Get.vi"("refnum name"="Hatch Kicker Solenoid") -> ("SolenoidDevRef"=w96:T6)  [unwired: 9 in, 1 out]
  n20 = call <vilib>:"WPI_SolenoidRefNum Registry Get.vi"("refnum name"="Hatch Retainer Solenoid") -> ("SolenoidDevRef"=w95:T6)  [unwired: 9 in, 1 out]
  n21 = call <vilib>:"WPI_DigitalInputRefNum Registry Get.vi"("refnum name"="Top Hatch Retainer Limit Switch") -> ("DigitalInputDevRef"=w30:T8)  [unwired: 9 in, 1 out]
  n22 = call <vilib>:"WPI_DigitalInputRefNum Registry Get.vi"("refnum name"="Bottom Hatch Retainer Limit Switch") -> ("DigitalInputDevRef"=w31:T8)  [unwired: 9 in, 1 out]
  n23 = call <vilib>:"WPI_MotorControlRefNum Registry Get.vi"("refnum name"="Hatch Retainer Motor") -> ("MotorControlDevRef"=w36:T1)  [unwired: 9 in, 1 out]
  n24 = call <vilib>:"WPI_MotorControlRefNum Registry Get.vi"("refnum name"="Hatch Collector Motor") -> ("MotorControlDevRef"=w74:T1)  [unwired: 9 in, 1 out]
  n25 = call <vilib>:"WPI_MotorControlRefNum Registry Get.vi"("refnum name"="HAB 3 Drive Module Motor") -> ("MotorControlDevRef"=w6:T1)  [unwired: 9 in, 1 out]
  n26 = call <vilib>:"WPI_JoystickRefNum Registry Get.vi"("refnum name"="Drive Joystick") -> ("JoystickDevRef"=w120:T9)  [unwired: 9 in, 1 out]
  n27 = call <vilib>:"WPI_JoystickRefNum Registry Get.vi"("refnum name"="Aux Joystick") -> ("JoystickDevRef"=w119:T9)  [unwired: 9 in, 1 out]
  n28 = call-poly <vilib>:"CTRE_Phoenix_MotorController_Get_Enhanced.vi"("PhoenixMotorControlDevRef"=w74) -> ("Quadrature Position"=w73:i32)  [unwired: 11 in, 3 out]
  n29 = call-poly <vilib>:"CTRE_Phoenix_MotorController_Get_Enhanced.vi"("PhoenixMotorControlDevRef"=w13) -> ("Quadrature Position"=w14:i32)  [unwired: 11 in, 3 out]
  n30 = disable-structure shown="Disabled" {
    disable-tunnel: [w132 _] -> w40
    frame Disabled {
      n31 = call <vilib>:"WPI_GyroRefNum Registry Get.vi"("refnum name"="Gyro") -> ("GyroDevRef"=w132:T23)  [unwired: 9 in, 1 out]
    }
    frame Enabled {
    }
  }
  n32 = global write "Robot Global Data.vi" "HAB Bk Spd Encoder Start Value"(w14) -> ()
  n33 = Bundle("Front Drive Motors"=w2, "HAB3DriveModuleMotorDevRef 2"="HAB3DriveModuleMotorDevRef 2", "DriveJoystickDevRef"="DriveJoystickDevRef", "AuxJoystickDevRef"="AuxJoystickDevRef", "Drive Axes"=w117, "Drive Buttons"=w116, "Drive POVs"=w115, "Aux Axes"=w114, "Aux Buttons"=w113, "Aux POVs"=w112, "Robot Mode"=w111, "Drive Motors"="Drive Motors", "Drive Axes Indexes"=w108, "Drive Button Indexes"=w106, "Joystick VS Vision Latch"=w105, "Vision States"=w104, "limelight"=w103, "Vision Track Mode Override"=w102, "T = Motion Profile, F = Percent Output"=w39, "Arcade Drive?"=w10, "Start Motion Profile?"=w9) -> (w121:T26)  [unwired: 1 in]
  n34 = Bundle By Name(cluster=w121, "HAB3DriveModuleMotorDevRef 2"=w6, "Front Drive Motors"=w109, "DriveJoystickDevRef"=w120, "AuxJoystickDevRef"=w119) -> (w118:T26)
  n35 = global write "Robot Global Data.vi" "Hatch Encoder Start Value"(w73) -> ()
  n36 = Bundle("TopRetainerSwitchDevRef"="TopRetainerSwitchDevRef", "BottomRetainerSwitchDevRef"="BottomRetainerSwitchDevRef", "HatchRetainerMotorDevRef"="HatchRetainerMotorDevRef", "LifterSolenoidDevRef"="LifterSolenoidDevRef", "DriveJoystickDevRef"="DriveJoystickDevRef", "KickerSolenoidDevRef"="KickerSolenoidDevRef", "RetainerSolenoidDevRef"="RetainerSolenoidDevRef", "AuxJoystickDevRef"="AuxJoystickDevRef", "HatchCollectorMotorDevRef"="HatchCollectorMotorDevRef", "Drive Axes"=w88, "Drive Buttons"=w87, "Drive POVs"=w86, "Aux Axes"=w85, "Aux Buttons"=w84, "Aux POVs"=w83, "Robot Mode"=w82, "Aux Joystick Indexes"=w78, "Aux Button Indexes"=w77, "Hatch Retainer Move Up/Down"=w76, "Hatch Collector Actual Angle"=w75, "Hatch Collector Wanted Angle"=w41, "Hatch Retainer States"=w29, "Hatch Kicking States"=w11) -> (w99:T27)  [unwired: 1 in]
  n37 = Bundle By Name(cluster=w99, "TopRetainerSwitchDevRef"=w30, "BottomRetainerSwitchDevRef"=w31, "HatchRetainerMotorDevRef"=w36, "HatchCollectorMotorDevRef"=w74, "DriveJoystickDevRef"=w79, "AuxJoystickDevRef"=w93, "KickerSolenoidDevRef"=w96, "RetainerSolenoidDevRef"=w95, "LifterSolenoidDevRef"=w71) -> (w89:T27)
  n38 = Bundle("BkSpdAdjusterMotorDevRef"="BkSpdAdjusterMotorDevRef", "HABAssisterSolenoidDevRef"="HABAssisterSolenoidDevRef", "Back HAB 3 Limit Switch"="Back HAB 3 Limit Switch", "Front HAB 3 Limit Switch"="Front HAB 3 Limit Switch", "HAB3DriveModuleMotorDevRef"="HAB3DriveModuleMotorDevRef", "DriveJoystickDevRef"="DriveJoystickDevRef", "AuxJoystickDevRef"="AuxJoystickDevRef", "HAB3FrontSolenoidDevRef"="HAB3FrontSolenoidDevRef", "HAB3BackSolenoidDevRef"="HAB3BackSolenoidDevRef", "Drive Axes"=w52, "Drive Buttons"=w51, "Drive POVs"=w50, "Aux Axes"=w49, "Aux Buttons"=w48, "Aux POVs"=w47, "Robot Mode"=w46, "Aux Joystick Indexes"=w45, "Aux Button Indexes"=w44, "Front Cylinders Latch"=w43, "Back Cylinders Latch"=w42, "Yaw"=w19, "Pitch"=w18, "Roll"=w17, "HAB Bk Spd Motor States"=w12) -> (w59:T28)  [unwired: 1 in]
  n39 = Bundle By Name(cluster=w59, "BkSpdAdjusterMotorDevRef"=w13, "HABAssisterSolenoidDevRef"=w20, "Front HAB 3 Limit Switch"=w24, "Back HAB 3 Limit Switch"=w23, "HAB3DriveModuleMotorDevRef"=w54, "DriveJoystickDevRef"=w55, "AuxJoystickDevRef"=w56, "HAB3FrontSolenoidDevRef"=w57, "HAB3BackSolenoidDevRef"=w58) -> (w53:T28)
  n40 = while {
    shift-right: [w217] -> _
    shift-left: w118 -> [w139]
    tunnel: w40 -> [w179]
    stop <- FALSE stop-if-true
    # "0 = Side-by-side stream\n1 = The secondary camera is placed\n       in the lower-right corner\n2 = The primary camera stream is\n       placed in the lower-right corner"
    # "converts encoder values\nto inches for auto if necessary"
    # "Parse our motion profile csv, each row is a trajectory point"
    # "Parse our motion profile csv, each row is a trajectory point"
    # "this allows us to exit the MP \neither if it finishes (since the\nMP control VI makes the\nlatch false when finished) \nor by pressing the cancel \nbutton"
    # "the Ys of the drive joysticks are \ninverted by default"
    n41 = disable-structure shown="Disabled" {
      disable-tunnel: w179 -> [w394 _]
      frame Disabled {
        n42 = call <vilib>:"WPI_GyroGetAngle.vi"("GyroDevRef"=w394) -> ("Angle"=w395:dbl)  [unwired: 6 in, 4 out]
        n43 = global write "Robot Global Data.vi" "Gyro"(w395) -> ()
      }
      frame Enabled {
      }
    }
    n44 = Unbundle By Name(w139) -> ("DriveJoystickDevRef"=w215:T9)
    n45 = Unbundle By Name(w139) -> ("AuxJoystickDevRef"=w214:T9)
    n46 = Unbundle By Name(w139) -> ("Robot Mode"=w213:T17)
    n47 = Unbundle By Name(w139) -> ("Robot Mode"=w138:T17)
    n48 = call <vilib>:"WPI_JoystickGetValues.vi"("JoystickDevRef"=w214) -> ("Buttons"=w206:bool[], "Axes"=w207:dbl[], "JoystickDevRef"=w208:T9, "POVs"=w205:i16[])  [unwired: 6 in, 1 out]
    n49 = call <vilib>:"WPI_JoystickGetValues.vi"("JoystickDevRef"=w215) -> ("Buttons"=w210:bool[], "Axes"=w212:dbl[], "JoystickDevRef"=w211:T9, "POVs"=w209:i16[])  [unwired: 6 in, 1 out]
    n50 = feedback #1() -> (w137:T17)  [unwired: 1 in]
    n51 = feedback-in #1(w138) -> ()
    n52 = case shown="\"Autonomous Enabled\"" w213 {
      tunnel: w139 -> [w412 w434 w440 w460 w466 w478 w490 w510 w516]
      tunnel: [w408 w420 w435 w447 w461 w473 w485 w497 w511] -> w178
      tunnel: w212 -> [_ w433 _ w458 _ _ _ w508 _]
      tunnel: w211 -> [_ w432 _ w459 _ _ _ w509 _]
      tunnel: w210 -> [_ w431 _ w457 _ _ _ w507 _]
      tunnel: w209 -> [_ w430 _ w456 _ _ _ w506 _]
      tunnel: w208 -> [_ w429 _ w455 _ _ _ w505 _]
      tunnel: w207 -> [_ w428 _ w454 _ _ _ w504 _]
      tunnel: w206 -> [_ w427 _ w453 _ _ _ w503 _]
      tunnel: w205 -> [_ w426 _ w452 _ _ _ w502 _]
      tunnel: w138 -> [_ w425 _ _ _ _ _ _ _]
      tunnel: w137 -> [_ w424 _ _ _ _ _ _ _]
      frame "Autonomous Disabled", Default {
        n53 = disable-structure shown="Enabled" {
          disable-tunnel: w412 -> [w414 w418]
          disable-tunnel: [w413 w417] -> w410
          frame Disabled {
            n54 = Bundle By Name(cluster=w414, "Joystick VS Vision Latch"=FALSE) -> (w413:T26)
          }
          frame Enabled {
            n55 = Bundle By Name(cluster=w418, "Vision States"=Vision_States."Ready") -> (w417:T26)
          }
        }
        n56 = Bundle By Name(cluster=w410, "Start Motion Profile?"=FALSE ("T = Motion Profile, F = Percent Output")) -> (w409:T26)
        n57 = Bundle By Name(cluster=w409, "T = Motion Profile, F = Percent Output"=FALSE) -> (w408:T26)
      }
      frame "Autonomous Enabled" {
        n58 = global read "Robot Global Data.vi" "Run the Motion Profile?"() -> (w419:bool)
        n59 = Not Equal?(x=w425, y=w424) -> (x != y?=w423:bool)
        n60 = Bundle By Name(cluster=w434, "DriveJoystickDevRef"=w432, "Drive Axes"=w433, "Drive Buttons"=w431, "Drive POVs"=w430, "AuxJoystickDevRef"=w429, "Aux Axes"=w428, "Aux Buttons"=w427, "Aux POVs"=w426) -> (w422:T26)
        n61 = Bundle By Name(cluster=w422, "Start Motion Profile?"=w423) -> (w421:T26)
        n62 = Bundle By Name(cluster=w421, "T = Motion Profile, F = Percent Output"=w419) -> (w420:T26)
      }
      frame "Teleop Disabled" {
        n63 = disable-structure shown="Enabled" {
          disable-tunnel: w440 -> [w442 w446]
          disable-tunnel: [w441 w445] -> w438
          frame Disabled {
            n64 = Bundle By Name(cluster=w442, "Joystick VS Vision Latch"=FALSE) -> (w441:T26)
          }
          frame Enabled {
            n65 = Bundle By Name(cluster=w446, "Vision States"=Vision_States."Ready") -> (w445:T26)
          }
        }
        n66 = Bundle By Name(cluster=w438, "Start Motion Profile?"=FALSE ("T = Motion Profile, F = Percent Output")) -> (w436:T26)
        n67 = Bundle By Name(cluster=w436, "T = Motion Profile, F = Percent Output"=FALSE) -> (w435:T26)
      }
      frame "Teleop Enabled" {
        n68 = Bundle By Name(cluster=w460, "DriveJoystickDevRef"=w459, "Drive Axes"=w458, "Drive Buttons"=w457, "Drive POVs"=w456, "AuxJoystickDevRef"=w455, "Aux Axes"=w454, "Aux Buttons"=w453, "Aux POVs"=w452) -> (w451:T26)
        n69 = Bundle By Name(cluster=w451, "Start Motion Profile?"=FALSE ("T = Motion Profile, F = Percent Output")) -> (w448:T26)
        n70 = Bundle By Name(cluster=w448, "T = Motion Profile, F = Percent Output"=FALSE) -> (w447:T26)
      }
      frame "Disconnected" {
        n71 = disable-structure shown="Enabled" {
          disable-tunnel: w466 -> [w468 w472]
          disable-tunnel: [w467 w471] -> w464
          frame Disabled {
            n72 = Bundle By Name(cluster=w468, "Joystick VS Vision Latch"=FALSE) -> (w467:T26)
          }
          frame Enabled {
            n73 = Bundle By Name(cluster=w472, "Vision States"=Vision_States."Ready") -> (w471:T26)
          }
        }
        n74 = Bundle By Name(cluster=w464, "Start Motion Profile?"=FALSE ("T = Motion Profile, F = Percent Output")) -> (w462:T26)
        n75 = Bundle By Name(cluster=w462, "T = Motion Profile, F = Percent Output"=FALSE) -> (w461:T26)
      }
      frame "Finish" {
        n76 = disable-structure shown="Enabled" {
          disable-tunnel: w478 -> [w480 w484]
          disable-tunnel: [w479 w483] -> w476
          frame Disabled {
            n77 = Bundle By Name(cluster=w480, "Joystick VS Vision Latch"=FALSE) -> (w479:T26)
          }
          frame Enabled {
            n78 = Bundle By Name(cluster=w484, "Vision States"=Vision_States."Ready") -> (w483:T26)
          }
        }
        n79 = Bundle By Name(cluster=w476, "Start Motion Profile?"=FALSE ("T = Motion Profile, F = Percent Output")) -> (w474:T26)
        n80 = Bundle By Name(cluster=w474, "T = Motion Profile, F = Percent Output"=FALSE) -> (w473:T26)
      }
      frame "Test Disabled" {
        n81 = disable-structure shown="Enabled" {
          disable-tunnel: w490 -> [w492 w496]
          disable-tunnel: [w491 w495] -> w488
          frame Disabled {
            n82 = Bundle By Name(cluster=w492, "Joystick VS Vision Latch"=FALSE) -> (w491:T26)
          }
          frame Enabled {
            n83 = Bundle By Name(cluster=w496, "Vision States"=Vision_States."Ready") -> (w495:T26)
          }
        }
        n84 = Bundle By Name(cluster=w488, "Start Motion Profile?"=FALSE ("T = Motion Profile, F = Percent Output")) -> (w486:T26)
        n85 = Bundle By Name(cluster=w486, "T = Motion Profile, F = Percent Output"=FALSE) -> (w485:T26)
      }
      frame "Test Enabled" {
        n86 = Bundle By Name(cluster=w510, "DriveJoystickDevRef"=w509, "Drive Axes"=w508, "Drive Buttons"=w507, "Drive POVs"=w506, "AuxJoystickDevRef"=w505, "Aux Axes"=w504, "Aux Buttons"=w503, "Aux POVs"=w502) -> (w500:T26)
        n87 = Bundle By Name(cluster=w500, "Start Motion Profile?"=FALSE ("T = Motion Profile, F = Percent Output")) -> (w498:T26)
        n88 = Bundle By Name(cluster=w498, "T = Motion Profile, F = Percent Output"=FALSE) -> (w497:T26)
      }
      frame "Emergency Stopped" {
        n89 = disable-structure shown="Enabled" {
          disable-tunnel: w516 -> [w518 w522]
          disable-tunnel: [w517 w521] -> w514
          frame Disabled {
            n90 = Bundle By Name(cluster=w518, "Joystick VS Vision Latch"=FALSE) -> (w517:T26)
          }
          frame Enabled {
            n91 = Bundle By Name(cluster=w522, "Vision States"=Vision_States."Ready") -> (w521:T26)
          }
        }
        n92 = Bundle By Name(cluster=w514, "Start Motion Profile?"=FALSE ("T = Motion Profile, F = Percent Output")) -> (w512:T26)
        n93 = Bundle By Name(cluster=w512, "T = Motion Profile, F = Percent Output"=FALSE) -> (w511:T26)
      }
    }
    n94 = Wait (ms)(milliseconds to wait=u32 50) -> ()  [unwired: 1 out]
    n95 = call-poly <vilib>:"NT Write Value.vi"("Numeric"=1, "Name"="/limelight/stream") -> ()  [unwired: 9 in, 1 out]
    n96 = disable-structure shown="Enabled" {
      disable-tunnel: w178 -> [w224 w227]
      disable-tunnel: [w222 w226] -> w177
      disable-tunnel: [w221 w225] -> w176
      frame Disabled {
        # "these numbers are the indexes of\nthe drive motors based on the\norder that they're opened in Begin"
        n97 = Unbundle By Name(w224) -> ("Drive Motors.Motors[]"=w223:T1[])
        n98 = Index Array(array=w223, index #1=2 ("index"), index #2=3 ("index")) -> (element #1=w222:T1, element #2=w221:T1)
      }
      frame Enabled {
        n99 = Unbundle By Name(w227) -> ("Front Drive Motors.FLDriveMotor"=w226:T1, "Front Drive Motors.FRDriveMotor"=w225:T1)
      }
    }
    n100 = Unbundle By Name(w178) -> ("Drive Buttons"=w184:bool[])
    n101 = Unbundle By Name(w178) -> ("Drive Button Indexes.A Button"=w201:i32)
    n102 = Unbundle By Name(w178) -> ("Drive Axes Indexes.Left X"=w186:i32, "Drive Axes Indexes.Left Y"=w187:i32, "Drive Axes Indexes.Right X"=w188:i32, "Drive Axes Indexes.Right Y"=w189:i32)
    n103 = Unbundle By Name(w178) -> ("Drive Buttons"=w183:bool[])
    n104 = Unbundle By Name(w178) -> ("Drive Button Indexes.LB Button"=w182:i32)
    n105 = Unbundle By Name(w178) -> ("Joystick VS Vision Latch"=w203:bool)
    n106 = Unbundle By Name(w178) -> ("Drive Axes"=w185:dbl[])
    n107 = global read "Robot Global Data.vi" "Robot Mode"() -> (w190:T17)
    n108 = Bundle By Name(cluster=w178, "Robot Mode"=w190) -> (w204:T26)
    n109 = Index Array(array=w184, index=w201) -> (element=w202:bool)
    n110 = global read "Robot Global Data.vi" "Which Robot?"() -> (w151:T30)
    n111 = Index Array(array=w185, index #1=w186, index #2=w187, index #3=w188, index #4=w189) -> (element #1=w194:dbl, element #2=w195:dbl, element #3=w196:dbl, element #4=w197:dbl)
    n112 = global read "Robot Global Data.vi" "Which Robot?"() -> (w157:T30)
    n113 = Index Array(array=w183, index=w182) -> (element=w180:bool)
    n114 = global read "Robot Global Data.vi" "Right Encoder Val. Initial"() -> (w158:dbl)
    n115 = global read "Robot Global Data.vi" "Left Encoder Val. Initial"() -> (w160:dbl)
    n116 = disable-structure shown="Enabled" {
      disable-tunnel: w202 -> [w398 w405]
      disable-tunnel: w203 -> [_ w403]
      disable-tunnel: w204 -> [_ w401]
      disable-tunnel: [_ w399] -> w181
      frame Disabled {
        n117 = feedback #2() -> (w397:bool)  [unwired: 1 in]
        n118 = feedback-in #2(w398) -> ()
        n119 = Greater?(x=w398, y=w397) -> (0:w396:bool)
        n120 = global write "Robot Global Data.vi" "Driver VS Vision Control"(w396) -> ()
      }
      frame Enabled {
        n121 = feedback #3() -> (w406:bool)  [unwired: 1 in]
        n122 = feedback-in #3(w405) -> ()
        n123 = Greater?(x=w405, y=w406) -> (0:w404:bool)
        n124 = Not(x=w403) -> (.not. x?=w402:bool)
        n125 = Select(t=w402, s=w404, f=w403) -> (s? t:f=w400:bool)
        n126 = global write "Robot Global Data.vi" "Driver VS Vision Control"(w400) -> ()
        n127 = Bundle By Name(cluster=w401, "Joystick VS Vision Latch"=w400) -> (w399:T26)
      }
    }
    n128 = call "Deadband.vi"("Input"=w194) -> ("Output"=w192:dbl)  [unwired: 10 in]
    n129 = call "Deadband.vi"("Input"=w195) -> ("Output"=w193:dbl)  [unwired: 10 in]
    n130 = call "Deadband.vi"("Input"=w196) -> ("Output"=w191:dbl)  [unwired: 10 in]
    n131 = call "Deadband.vi"("Input"=w197) -> ("Output"=w198:dbl)  [unwired: 10 in]
    n132 = call-poly <vilib>:"CTRE_Phoenix_MotorController_Get_Enhanced.vi"("PhoenixMotorControlDevRef"=w177) -> ("Quadrature Position"=w161:i32)  [unwired: 11 in, 3 out]
    n133 = call-poly <vilib>:"CTRE_Phoenix_MotorController_Get_Enhanced.vi"("PhoenixMotorControlDevRef"=w176) -> ("Quadrature Position"=w159:i32)  [unwired: 11 in, 3 out]
    n134 = Negate(x=w193) -> (-x=w199:dbl)
    n135 = Negate(x=w198) -> (-x=w200:dbl)
    n136 = global write "Robot Global Data.vi" "Left Drive Joystick X"(w192) -> ()
    n137 = global write "Robot Global Data.vi" "Right Drive Joystick X"(w191) -> ()
    n138 = case shown="\"Competition Bot\", Default" w151 {
      tunnel: [w229 w231 w233] -> w150
      tunnel: [w228 w230 w232] -> w149
      frame "Competition Bot", Default {
        w228 = 18069  # Change in Encoder
        w229 = 84  # Change in Distance (inches)
      }
      frame "Practice Bot" {
        w230 = 0  # Change in Encoder
        w231 = 0  # Change in Distance (inches)
      }
      frame "Code Bot" {
        w232 = 0  # Change in Encoder
        w233 = 0  # Change in Distance (inches)
      }
    }
    n139 = global write "Robot Global Data.vi" "Right Drive Joystick Y"(w200) -> ()
    n140 = global write "Robot Global Data.vi" "Left Drive Joystick Y"(w199) -> ()
    n141 = case shown="\"Competition Bot\", Default" w157 {
      tunnel: [w235 w237 w239] -> w156
      tunnel: [w234 w236 w238] -> w155
      frame "Competition Bot", Default {
        w234 = 17996  # Change in Encoder
        w235 = 84  # Change in Distance (inches)
      }
      frame "Practice Bot" {
        w236 = 0  # Change in Encoder
        w237 = 0  # Change in Distance (inches)
      }
      frame "Code Bot" {
        w238 = 0  # Change in Encoder
        w239 = 0  # Change in Distance (inches)
      }
    }
    n142 = Subtract(x=w161, y=w160) -> (x-y=w153:dbl)
    n143 = Subtract(x=w159, y=w158) -> (x-y=w147:dbl)
    n144 = Bundle By Name(cluster=w181, "Vision Track Mode Override"=w180) -> (w136:T26)
    n145 = global write "Robot Global Data.vi" "Right Encoder in Enc. Vals"(w147) -> ()
    n146 = global write "Robot Global Data.vi" "Left Encoder in Enc. Vals"(w153) -> ()
    n147 = Divide(x=w150, y=w149) -> (x/y=w146:dbl)
    n148 = Divide(x=w156, y=w155) -> (x/y=w154:dbl)
    n149 = Multiply(x=w154, y=w153) -> (x*y=w152:dbl)
    n150 = Multiply(x=w147, y=w146) -> (x*y=w148:dbl)
    n151 = global write "Robot Global Data.vi" "Left Encoder in Inches"(w152) -> ()
    n152 = global write "Robot Global Data.vi" "Right Encoder in Inches"(w148) -> ()
    n153 = disable-structure shown="Enabled" {
      disable-tunnel: w136 -> [w289 w296]
      frame Disabled {
        n154 = Unbundle By Name(w289) -> ("Drive Button Indexes.RB Button"=w288:i32)
        n155 = Unbundle By Name(w289) -> ("Drive Buttons"=w287:bool[])
        n156 = Unbundle By Name(w289) -> ("T = Motion Profile, F = Percent Output"=w282:bool)
        n157 = Index Array(array=w287, index=w288) -> (element=w285:bool)
        n158 = feedback #4() -> (w286:bool)  [unwired: 1 in]
        n159 = feedback-in #4(w285) -> ()
        n160 = Greater?(x=w285, y=w286) -> (0:w284:bool)
        n161 = Not(x=w282) -> (.not. x?=w283:bool)
        n162 = Select(t=w283, s=w284, f=w282) -> ()  [unwired: 1 out]
      }
      frame Enabled {
        n163 = Unbundle By Name(w296) -> ("Drive Button Indexes.Y Button"=w298:i32)
        n164 = Unbundle By Name(w296) -> ("Drive Buttons"=w297:bool[])
        n165 = global read "Robot Global Data.vi" "Cancel the Motion Profile?"() -> (w290:bool)
        n166 = Index Array(array=w297, index=w298) -> (element=w292:bool)
        n167 = feedback #5() -> (w295:bool)  [unwired: 1 in]
        n168 = feedback-in #5(w292) -> ()
        n169 = Greater?(x=w292, y=w295) -> (0:w294:bool)
        n170 = Not(x=w290) -> (.not. x?=w293:bool)
        n171 = Select(t=w293, s=w294, f=w290) -> (s? t:f=w291:bool)
        n172 = global write "Robot Global Data.vi" "Cancel the Motion Profile?"(w291) -> ()
      }
    }
    n173 = Unbundle By Name(w136) -> ("Drive Button Indexes.RB Button"=w143:i32)
    n174 = Unbundle By Name(w136) -> ("Drive Buttons"=w142:bool[])
    n175 = Index Array(array=w142, index=w143) -> (element=w141:bool)
    n176 = Bundle By Name(cluster=w136, "Arcade Drive?"=w141) -> (w135:T26)
    n177 = call "RIGHT Motion Profile Traj Points Array.vi"("Read = false, Write = true"=FALSE) -> ("traj. points array out"=w162:dbl[][])  [unwired: 10 in]
    "Right Traj. Pts Array" <- w162
    n178 = call "LEFT Motion Profile Traj Points Array.vi"("Read = false, Write = true"=FALSE) -> ("traj. points array out"=w169:dbl[][])  [unwired: 10 in]
    "Left Traj. Pts Array" <- w169
    n179 = for {
      N -> [w253]
      tunnel: w162 -> [w259] mode=indexing
      tunnel: [w249] -> w168 mode=indexing
      i -> [w252]
      w258 = 0.0 ("Arbitrary Feed Forward")
      # "Convert profile units to talon units"
      n180 = Decrement(x=w253) -> (x-1=w254:i32)
      n181 = Equal?(x=w254, y=w252) -> (x = y?=w255:bool)
      n182 = Equal To 0?(x=w252) -> (x = 0?=w251:bool)
      n183 = Index Array(array=w259) -> (element #1=w247:dbl, element #2=w241:dbl, element #3=w248:dbl)  [unwired: 3 in]
      n184 = Multiply(x=4096.0, y=w241) -> (x*y=w243:dbl)
      n185 = Multiply(x=4096.0, y=w247) -> (x*y=w245:dbl)
      n186 = Divide(x=w243, y=10.0) -> (x/y=w240:dbl)
      n187 = Bundle By Name(cluster=T29 {"Position"=0.0, "Velocity"=0.0, "Arbitrary Feed Forward"=0.0, "Auxiliary Position"=0.0, "Auxiliary Velocity"=0.0, "Auxiliary Arbitrary Feed Forward"=0.0, "Profile Slot Select"=0, "Auxiliary Profile Slot Select"=0, "isLastPoint?"=FALSE, "Zero Position?"=FALSE, "durationMs"=0, "Use Aux PID?"=FALSE} ("Trajectory Point"), "Position"=w245, "Velocity"=w240, "Arbitrary Feed Forward"=w258, "Auxiliary Position"=w258, "Auxiliary Velocity"=w258, "Auxiliary Arbitrary Feed Forward"=w258, "Profile Slot Select"=0, "Auxiliary Profile Slot Select"=1, "isLastPoint?"=w255, "Zero Position?"=w251, "durationMs"=w248, "Use Aux PID?"=FALSE) -> (w249:T29)
    }
    n188 = for {
      N -> [w274]
      tunnel: w169 -> [w280] mode=indexing
      tunnel: [w270] -> w175 mode=indexing
      i -> [w273]
      w279 = 0.0 ("Arbitrary Feed Forward")
      # "Convert profile units to talon units"
      n189 = Decrement(x=w274) -> (x-1=w275:i32)
      n190 = Equal?(x=w275, y=w273) -> (x = y?=w276:bool)
      n191 = Equal To 0?(x=w273) -> (x = 0?=w272:bool)
      n192 = Index Array(array=w280) -> (element #1=w268:dbl, element #2=w262:dbl, element #3=w269:dbl)  [unwired: 3 in]
      n193 = Multiply(x=4096.0, y=w262) -> (x*y=w264:dbl)
      n194 = Multiply(x=4096.0, y=w268) -> (x*y=w266:dbl)
      n195 = Divide(x=w264, y=10.0) -> (x/y=w261:dbl)
      n196 = Bundle By Name(cluster=T29 {"Position"=0.0, "Velocity"=0.0, "Arbitrary Feed Forward"=0.0, "Auxiliary Position"=0.0, "Auxiliary Velocity"=0.0, "Auxiliary Arbitrary Feed Forward"=0.0, "Profile Slot Select"=0, "Auxiliary Profile Slot Select"=0, "isLastPoint?"=FALSE, "Zero Position?"=FALSE, "durationMs"=0, "Use Aux PID?"=FALSE} ("Trajectory Point"), "Position"=w266, "Velocity"=w261, "Arbitrary Feed Forward"=w279, "Auxiliary Position"=w279, "Auxiliary Velocity"=w279, "Auxiliary Arbitrary Feed Forward"=w279, "Profile Slot Select"=0, "Auxiliary Profile Slot Select"=1, "isLastPoint?"=w276, "Zero Position?"=w272, "durationMs"=w269, "Use Aux PID?"=FALSE) -> (w270:T29)
    }
    n197 = call <vilib>:"CTRE_Phoenix_MotorControl_BufferedTrajectoryPointStream_Open.vi"() -> ("BufferedTrajectoryPointStream_DevRef"=w167:T31)  [unwired: 10 in, 1 out]
    n198 = call <vilib>:"CTRE_Phoenix_MotorControl_BufferedTrajectoryPointStream_Open.vi"() -> ("BufferedTrajectoryPointStream_DevRef"=w174:T31)  [unwired: 10 in, 1 out]
    n199 = call-poly <vilib>:"CTRE_Phoenix_MotorControl_BufferedTrajectoryPointStream_Write.vi"("Motion Profile Trajectory Point Array"=w168, "BufferedTrajectoryPointStream_DevRef"=w167) -> ("error out"=w165:errorcluster, "BufferedTrajectoryPointStream_DevRef"=w166:T31)  [unwired: 8 in]
    n200 = call-poly <vilib>:"CTRE_Phoenix_MotorControl_BufferedTrajectoryPointStream_Write.vi"("Motion Profile Trajectory Point Array"=w175, "BufferedTrajectoryPointStream_DevRef"=w174) -> ("error out"=w172:errorcluster, "BufferedTrajectoryPointStream_DevRef"=w173:T31)  [unwired: 8 in]
    n201 = call <vilib>:"CTRE_Phoenix_MotorControl_BufferedTrajectoryPointStream_SetDeviceReference.vi"("error in (no error)"=w165, "refnum name"="right_mpStream", "BufferedTrajectoryPointStream_DevRef"=w166) -> ()  [unwired: 7 in, 2 out]
    n202 = call <vilib>:"CTRE_Phoenix_MotorControl_BufferedTrajectoryPointStream_SetDeviceReference.vi"("error in (no error)"=w172, "refnum name"="left_mpStream", "BufferedTrajectoryPointStream_DevRef"=w173) -> ()  [unwired: 7 in, 2 out]
    n203 = Unbundle By Name(w135) -> ("T = Motion Profile, F = Percent Output"=w140:bool)
    n204 = Unbundle By Name(w135) -> ("Start Motion Profile?"=w134:bool)
    n205 = case shown="True" w140 {
      tunnel: [w300 w392] -> w217
      tunnel: w135 -> [w299 w393]
      tunnel: w134 -> [_ w391]
      frame False {
        n206 = disable-structure shown="Enabled" {
          disable-tunnel: [w316 w336] -> w300
          disable-tunnel: w299 -> [w308 w322]
          frame Enabled {
            # "Vision and Joystick Control for Drive Train"
            # "for ease of testing\nfor programmers"
            # "1 = force off\n3 = force on"
            # "0 = vision processor\n1 = driver camera settings"
            n207 = Unbundle By Name(w308) -> ("Joystick VS Vision Latch"=w312:bool)
            n208 = Unbundle By Name(w308) -> ("Vision Track Mode Override"=w304:bool)
            n209 = Select(t=3, s=w312, f=1) -> (s? t:f=w303:i32)
            n210 = Select(t=0, s=w312, f=1) -> (s? t:f=w307:i32)
            n211 = Select(t=3, s=w304, f=w303) -> (s? t:f=w302:i32)
            n212 = Select(t=0, s=w304, f=w307) -> (s? t:f=w305:i32)
            n213 = case shown="False" w312 {
              tunnel: w308 -> [w317 w319]
              tunnel: [w317 w320] -> w316
              frame False {
                n214 = Unbundle By Name(w317) -> ("Arcade Drive?"=w318:bool)
                n215 = call "Joystick Drive Control.vi"("Arcade Drive?"=w318, "Cluster In"=w317) -> ()  [unwired: 10 in]
              }
              frame True {
                n216 = call "Vision Tracking Drive Control.vi"("Cluster In"=w319) -> ("Cluster Out"=w320:T26)  [unwired: 10 in]
              }
            }
            n217 = call-poly <vilib>:"NT Write Value.vi"("Numeric"=w305, "Name"="/limelight/camMode") -> ()  [unwired: 9 in, 1 out]
            n218 = call-poly <vilib>:"NT Write Value.vi"("Numeric"=w302, "Name"="/limelight/ledMode") -> ()  [unwired: 9 in, 1 out]
          }
          frame Disabled {
            n219 = call-poly <vilib>:"NT Read Value.vi"("Name"="/limelight/tx") -> ("Numeric"=w330:dbl)  [unwired: 9 in, 1 out]
            n220 = call-poly <vilib>:"NT Read Value.vi"("Name"="/limelight/ty") -> ("Numeric"=w329:dbl)  [unwired: 9 in, 1 out]
            n221 = call-poly <vilib>:"NT Read Value.vi"("Name"="/limelight/ta") -> ("Numeric"=w328:dbl)  [unwired: 9 in, 1 out]
            n222 = call-poly <vilib>:"NT Read Value.vi"("Name"="/limelight/ts") -> ("Numeric"=w327:dbl)  [unwired: 9 in, 1 out]
            n223 = call-poly <vilib>:"NT Read Value.vi"("Name"="/limelight/tshort") -> ("Numeric"=w324:dbl)  [unwired: 9 in, 1 out]
            n224 = call-poly <vilib>:"NT Read Value.vi"("Name"="/limelight/tlong") -> ("Numeric"=w323:dbl)  [unwired: 9 in, 1 out]
            n225 = Bundle By Name(cluster=w322, "limelight.offsetAngle H"=w330, "limelight.offsetAngle V"=w329, "limelight.area"=w328, "limelight.skew"=w327, "limelight.shortest side (pxls)"=w324, "limelight.longest side (pxls)"=w323) -> (w321:T26)
            n226 = Unbundle By Name(w321) -> ("Vision States"=w338:T19)
            n227 = case shown="\"Ready\", Default" w338 {
              tunnel: [w339 w354 w372] -> w337
              tunnel: w321 -> [w339 w354 w372]
              tunnel: [w348 w355 w368] -> w335
              frame "Ready", Default {
                # "should have created a \nboolean in the cluster \ninstead of just pulling\nthe A button"
                # "the Ys of the drive joysticks are \ninverted by default"
                n228 = Unbundle By Name(w339) -> ("Drive Button Indexes.A Button"=w353:i32)
                n229 = Unbundle By Name(w339) -> ("Drive Buttons"=w352:bool[])
                n230 = Unbundle By Name(w339) -> ("Drive Motors"=w347:T11, "Drive Axes"=w346:dbl[], "Drive Axes Indexes.Left Y"=w345:i32, "Drive Axes Indexes.Right Y"=w344:i32)
                n231 = Index Array(array=w352, index=w353) -> (element=w351:bool)
                n232 = Index Array(array=w346, index #1=w345, index #2=w344) -> (element #1=w343:dbl, element #2=w342:dbl)
                n233 = Negate(x=w343) -> (-x=w340:dbl)
                n234 = Negate(x=w342) -> (-x=w341:dbl)
                n235 = Select(t=Vision_States."Forward Until Target at Edge" ("Vision States"), s=w351, f=Vision_States."Ready" ("Vision States")) -> (s? t:f=w348:T19)
                n236 = call <vilib>:"WPI_RobotDriveTankDrive.vi"("Right axis value"=w341, "Left axis value"=w340, "RobotDriveDevRef"=w347) -> ()  [unwired: 6 in, 3 out]
              }
              frame "Forward Until Target at Edge" {
                n237 = Unbundle By Name(w354) -> ("limelight.offsetAngle H"=w359:dbl)
                n238 = Less?(x=w359, y=-26) -> (x < y?=w357:bool)
                n239 = Greater?(x=w359, y=14) -> (0:w358:bool)
                n240 = Or(x=w358, y=w357) -> (x .or. y?=w356:bool)
                n241 = case shown="False" w356 {
                  tunnel: [Vision_States."Forward Until Target at Edge" ("Vision States") Vision_States."Vision Track" ("Vision States")] -> w355
                  tunnel: w354 -> [w365 _]
                  frame False {
                    w363 = 0.35
                    n242 = Unbundle By Name(w365) -> ("Drive Motors"=w364:T11)
                    n243 = call <vilib>:"WPI_RobotDriveTankDrive.vi"("Right axis value"=w363, "Left axis value"=w363, "RobotDriveDevRef"=w364) -> ()  [unwired: 6 in, 3 out]
                  }
                  frame True {
                  }
                }
              }
              frame "Vision Track" {
                w375 = 0.5 ("t")
                w374 = 1.5
                # "this is the target area for\nwhen to stop driving \ntoward target (10 here \nwould means 10% of \nlimelight feed)"
                # "Hori. offset scaled down to\nbe a reasonable drive speed\ncoefficient (e.g. if this number\nis 0.01, 10deg offset to the \nleft would make right train \nrun at 110% and left train \nat 90%)"
                # "0deg offset = speed \nadjustment coefficient of 1"
                n244 = Unbundle By Name(w372) -> ("limelight.area"=w380:dbl, "limelight.offsetAngle H"=w388:dbl)
                n245 = Multiply(x=w388, y=0.03) -> (x*y=w377:dbl)
                n246 = Unbundle By Name(w372) -> ("Drive Motors"=w373:T11)
                n247 = Add(x=1.0, y=w377) -> (x+y=w383:dbl)
                n248 = Subtract(x=1.0, y=w377) -> (x-y=w376:dbl)
                n249 = Less?(x=w380, y=w374) -> (x < y?=w371:bool)
                n250 = Less?(x=w380, y=w374) -> (x < y?=w384:bool)
                n251 = Select(t=w375, s=w371, f=0.0) -> (s? t:f=w389:dbl)
                n252 = Select(t=w375, s=w384, f=0.0) -> (s? t:f=w381:dbl)
                n253 = Multiply(x=w389, y=w383) -> (x*y=w386:dbl)
                n254 = Multiply(x=w376, y=w381) -> (x*y=w379:dbl)
                n255 = Not(x=w371) -> (.not. x?=w367:bool)
                n256 = call <vilib>:"WPI_RobotDriveTankDrive.vi"("Right axis value"=w379, "Left axis value"=w386, "RobotDriveDevRef"=w373) -> ()  [unwired: 6 in, 3 out]
                n257 = Select(t=Vision_States."Ready" ("Vision States"), s=w367, f=Vision_States."Vision Track" ("Vision States")) -> (s? t:f=w368:T19)
              }
            }
            n258 = Bundle By Name(cluster=w337, "Vision States"=w335) -> (w336:T26)
          }
        }
      }
      frame True {
        # "left MP will control when the motion profile ends"
        # "Motion Profile Control for Drive Train"
        n259 = call "Motion Profile Left Drive Control.vi"("Start Motion Profile?"=w391, "Cluster In"=w393) -> ("Cluster Out"=w392:T26)  [unwired: 9 in]
        n260 = call "Motion Profile Right Drive Control.vi"("Start Motion Profile?"=w391, "Cluster In"=w393) -> ()  [unwired: 9 in, 1 out]
      }
    }
  }
  n261 = while {
    shift-right: [w526] -> _
    shift-left: w89 -> [w572]
    stop <- FALSE stop-if-true
    # "this chunk of code \ncontrols the wanted\nangle of the collector\nusing a joystick and\n2 angle presets"
    # "use this to scale the rate at which the\nwanted angle changes based on the joystick"
    # "we use this to set the\n\"0\" of the encoder to be \nwherever it is when the code\nis run (or the robot is turned\non in the case of \nhard-deployed code)"
    # "this chunk of code \nconverts the encoder\n values into angles"
    n262 = Unbundle By Name(w572) -> ("DriveJoystickDevRef"=w583:T9)
    n263 = Unbundle By Name(w572) -> ("AuxJoystickDevRef"=w582:T9)
    n264 = Unbundle By Name(w572) -> ("Robot Mode"=w581:T17)
    n265 = Wait (ms)(milliseconds to wait=u32 50) -> ()  [unwired: 1 out]
    n266 = call <vilib>:"WPI_JoystickGetValues.vi"("JoystickDevRef"=w582) -> ("Buttons"=w574:bool[], "Axes"=w575:dbl[], "JoystickDevRef"=w576:T9, "POVs"=w573:i16[])  [unwired: 6 in, 1 out]
    n267 = call <vilib>:"WPI_JoystickGetValues.vi"("JoystickDevRef"=w583) -> ("Buttons"=w578:bool[], "Axes"=w580:dbl[], "JoystickDevRef"=w579:T9, "POVs"=w577:i16[])  [unwired: 6 in, 1 out]
    n268 = case shown="\"Teleop Enabled\"" w581 {
      tunnel: w572 -> [w801 w811 w812 w813 w823 w824 w825 w835 w836]
      tunnel: [w801 w802 w812 w814 w823 w824 w825 w826 w836] -> w549
      tunnel: w580 -> [_ w810 _ w821 _ _ _ w833 _]
      tunnel: w579 -> [_ w809 _ w822 _ _ _ w834 _]
      tunnel: w578 -> [_ w808 _ w820 _ _ _ w832 _]
      tunnel: w577 -> [_ w807 _ w819 _ _ _ w831 _]
      tunnel: w576 -> [_ w806 _ w818 _ _ _ w830 _]
      tunnel: w575 -> [_ w805 _ w817 _ _ _ w829 _]
      tunnel: w574 -> [_ w804 _ w816 _ _ _ w828 _]
      tunnel: w573 -> [_ w803 _ w815 _ _ _ w827 _]
      frame "Autonomous Disabled", Default {
      }
      frame "Autonomous Enabled" {
        n269 = Bundle By Name(cluster=w811, "DriveJoystickDevRef"=w809, "Drive Axes"=w810, "Drive Buttons"=w808, "Drive POVs"=w807, "AuxJoystickDevRef"=w806, "Aux Axes"=w805, "Aux Buttons"=w804, "Aux POVs"=w803) -> (w802:T27)
      }
      frame "Teleop Disabled" {
      }
      frame "Teleop Enabled" {
        n270 = Bundle By Name(cluster=w813, "DriveJoystickDevRef"=w822, "Drive Axes"=w821, "Drive Buttons"=w820, "Drive POVs"=w819, "AuxJoystickDevRef"=w818, "Aux Axes"=w817, "Aux Buttons"=w816, "Aux POVs"=w815) -> (w814:T27)
      }
      frame "Disconnected" {
      }
      frame "Finish" {
      }
      frame "Test Disabled" {
      }
      frame "Test Enabled" {
        n271 = Bundle By Name(cluster=w835, "DriveJoystickDevRef"=w834, "Drive Axes"=w833, "Drive Buttons"=w832, "Drive POVs"=w831, "AuxJoystickDevRef"=w830, "Aux Axes"=w829, "Aux Buttons"=w828, "Aux POVs"=w827) -> (w826:T27)
      }
      frame "Emergency Stopped" {
      }
    }
    n272 = Unbundle By Name(w549) -> ("Aux Button Indexes.RB Button"=w547:i32)
    n273 = Unbundle By Name(w549) -> ("Aux Button Indexes.RT Button"=w546:i32)
    n274 = Unbundle By Name(w549) -> ("Aux Joystick Indexes.Right Y"=w556:i32)
    n275 = Unbundle By Name(w549) -> ("Aux Button Indexes.LT Button"=w570:i32)
    n276 = Unbundle By Name(w549) -> ("Aux Axes"=w557:dbl[])
    n277 = Unbundle By Name(w549) -> ("Aux Buttons"=w548:bool[])
    n278 = Unbundle By Name(w549) -> ("Aux Buttons"=w569:bool[])
    n279 = Unbundle By Name(w549) -> ("Hatch Collector Wanted Angle"=w554:dbl)
    n280 = Unbundle By Name(w549) -> ("Hatch Retainer Move Up/Down"=w566:bool)
    n281 = Unbundle By Name(w549) -> ("HatchCollectorMotorDevRef"=w563:T1)
    n282 = global read "Robot Global Data.vi" "Hatch Encoder Start Value"() -> (w558:dbl)
    n283 = global read "Robot Global Data.vi" "Robot Mode"() -> (w571:T17)
    n284 = global read "Robot Global Data.vi" "Which Robot?"() -> (w534:T30)
    n285 = Bundle By Name(cluster=w549, "Robot Mode"=w571) -> (w568:T27)
    n286 = call-poly <vilib>:"CTRE_Phoenix_MotorController_Get_Enhanced.vi"("PhoenixMotorControlDevRef"=w563) -> ("Quadrature Position"=w561:i32)  [unwired: 11 in, 3 out]
    n287 = Index Array(array=w557, index=w556) -> (element=w540:dbl)
    n288 = Index Array(array=w569, index=w570) -> (element=w567:bool)
    n289 = Index Array(array=w548, index #1=w547, index #2=w546) -> (element #1=w543:bool, element #2=w544:bool)
    n290 = call "Deadband.vi"("Input"=w540) -> ("Output"=w538:dbl)  [unwired: 10 in]
    n291 = disable-structure shown="Enabled" {
      disable-tunnel: w567 -> [w756 w760]
      disable-tunnel: w566 -> [w753 _]
      disable-tunnel: [w752 w759] -> w565
      frame Disabled {
        n292 = feedback #6() -> (w757:bool)  [unwired: 1 in]
        n293 = feedback-in #6(w756) -> ()
        n294 = Greater?(x=w756, y=w757) -> (0:w755:bool)
        n295 = Not(x=w753) -> (.not. x?=w754:bool)
        n296 = Select(t=w754, s=w755, f=w753) -> (s? t:f=w752:bool)
      }
      frame Enabled {
        n297 = feedback #7() -> (w758:bool)  [unwired: 1 in]
        n298 = feedback-in #7(w760) -> ()
        n299 = Greater?(x=w760, y=w758) -> (0:w759:bool)
      }
    }
    n300 = case shown="\"Competition Bot\", Default" w534 {
      tunnel: [w776 w785 w794] -> w562
      tunnel: w561 -> [w774 w784 w793]
      tunnel: w558 -> [w775 w783 w792]
      frame "Competition Bot", Default {
        # "range of \ndegrees"
        # "enc. val at\n\"max out\"\ndeg IRL"
        # "enc. val at\n\"max in\"\ndeg IRL"
        n301 = Subtract(x=w774, y=w775) -> (x-y=w777:dbl)
        n302 = Subtract(x=1047.0, y=46.0) -> (x-y=w781:dbl)
        n303 = Divide(x=97.0, y=w781) -> (x/y=w779:dbl)
        n304 = Multiply(x=w779, y=w777) -> (x*y=w776:dbl)
      }
      frame "Practice Bot" {
        # "range of \ndegrees"
        # "enc. val at\n\"max out\"\ndeg IRL"
        # "enc. val at\n\"max in\"\ndeg IRL"
        n305 = Subtract(x=w784, y=w783) -> (x-y=w786:dbl)
        n306 = Subtract(x=1050.0, y=34.0) -> (x-y=w790:dbl)
        n307 = Divide(x=90.0, y=w790) -> (x/y=w788:dbl)
        n308 = Multiply(x=w788, y=w786) -> (x*y=w785:dbl)
      }
      frame "Code Bot" {
        # "range of \ndegrees"
        # "enc. val at\n\"max out\"\ndeg IRL"
        # "enc. val at\n\"max in\"\ndeg IRL"
        n309 = Subtract(x=w793, y=w792) -> (x-y=w795:dbl)
        n310 = Subtract(x=1050.0, y=34.0) -> (x-y=w799:dbl)
        n311 = Divide(x=90.0, y=w799) -> (x/y=w797:dbl)
        n312 = Multiply(x=w797, y=w795) -> (x*y=w794:dbl)
      }
    }
    n313 = Add(x=w554, y=w538) -> (x+y=w553:dbl)
    n314 = Or(x=w543, y=w544) -> (x .or. y?=w545:bool)
    n315 = Multiply(x=1.0, y=w553) -> (x*y=w550:dbl)
    n316 = case shown="True" w545 {
      tunnel: [w769 w770] -> w551
      tunnel: w550 -> [w769 _]
      tunnel: w543 -> [_ w771]
      frame False {
        # "neither \npreset,\nJS controls\nwanted angle"
      }
      frame True {
        n317 = case shown="True" w771 {
          tunnel: [80.0 7.0] -> w770
          frame False {
            # "preset \nfor \nhovering\nto use \ndustpan"
          }
          frame True {
            # "preset\nfor \nvertical"
          }
        }
      }
    }
    n318 = global read "Robot Global Data.vi" "Which Robot?"() -> (w533:T30)
    n319 = case shown="\"Competition Bot\", Default" w533 {
      tunnel: [97.0 99.0 90.0] -> w532
      frame "Competition Bot", Default {
        # "max deg"
      }
      frame "Practice Bot" {
        # "max deg"
      }
      frame "Code Bot" {
        # "max deg"
      }
    }
    n320 = In Range and Coerce(upper limit=w532, x=w551, lower limit=0.0) -> (coerced(x)=w542:dbl)  [unwired: 1 out]
    n321 = Bundle By Name(cluster=w568, "Hatch Retainer Move Up/Down"=w565) -> (w564:T27)
    n322 = Bundle By Name(cluster=w564, "Hatch Collector Actual Angle"=w562) -> (w555:T27)
    n323 = Bundle By Name(cluster=w555, "Hatch Collector Wanted Angle"=w542) -> (w527:T27)
    n324 = disable-structure shown="Enabled" {
      disable-tunnel: [w676 w699] -> w528
      disable-tunnel: w527 -> [w674 w709]
      disable-tunnel: w527 -> [w673 w702]
      frame Disabled {
        # "only let kickers kick\nif the hatch retainer\nis fully down"
        # "if kick button was just pressed, go\ndown. Otherwise, keep the states\nas they are"
        n325 = Unbundle By Name(w673) -> ("KickerSolenoidDevRef"=w691:T6)
        n326 = Unbundle By Name(w673) -> ("Hatch Retainer States"=w678:T14)
        n327 = Unbundle By Name(w673) -> ("Aux Button Indexes.LB Button"=w689:i32)
        n328 = Unbundle By Name(w673) -> ("Aux Buttons"=w690:bool[])
        n329 = global read "Robot Global Data.vi" "Kick Hatch in Auto"() -> (w684:bool)
        n330 = case shown="\"Fully Down (not retained)\", Default" w678 {
          tunnel: [TRUE FALSE FALSE FALSE] -> w682
          frame "Fully Down (not retained)", Default {
          }
          frame "Going Up" {
          }
          frame "Fully Up (retained)" {
          }
          frame "Going Down" {
          }
        }
        n331 = Index Array(array=w690, index=w689) -> (element=w685:bool)
        n332 = Or(x=w685, y=w684) -> (x .or. y?=w680:bool)
        n333 = And(x=w680, y=w682) -> (x .and. y?=w683:bool)
        n334 = feedback #8() -> (w681:bool)  [unwired: 1 in]
        n335 = feedback-in #8(w680) -> ()
        n336 = Select(t=WPI_SolenoidValue."On" ("Value"), s=w683, f=WPI_SolenoidValue."Off" ("Value")) -> (s? t:f=w686:T32)
        n337 = Greater?(x=w680, y=w681) -> (0:w679:bool)
        n338 = call-poly <vilib>:"WPI_SolenoidSet.vi"("Value"=w686, "SolenoidDevRef"=w691) -> ()  [unwired: 8 in, 2 out]
        n339 = Select(t=Hatch_Retainer_States."Going Down" ("Hatch Retainer States"), s=w679, f=w678) -> (s? t:f=w677:T14)
        n340 = Bundle By Name(cluster=w674, "Hatch Retainer States"=w677) -> (w676:T27)
      }
      frame Enabled {
        n341 = Unbundle By Name(w702) -> ("Aux Button Indexes.LB Button"=w707:i32)
        n342 = Unbundle By Name(w702) -> ("Hatch Kicking States"=w697:T12)
        n343 = Unbundle By Name(w702) -> ("Aux Buttons"=w708:bool[])
        n344 = Unbundle By Name(w702) -> ("Hatch Retainer States"=w701:T14)
        n345 = Unbundle By Name(w702) -> ("KickerSolenoidDevRef"=w706:T6)
        n346 = feedback #9() -> (w696:T12)  [unwired: 1 in]
        n347 = feedback-in #9(w697) -> ()
        n348 = Index Array(array=w708, index=w707) -> (element=w703:bool)
        n349 = case shown="\"Kick Hatch\"" w697 {
          selector: w697 -> [_ _ w734]
          tunnel: [WPI_SolenoidValue."Off" ("Value") WPI_SolenoidValue."Off" ("Value") w731] -> w705
          tunnel: [w711 w718 w735] -> w704
          tunnel: w703 -> [w714 _ _]
          tunnel: w701 -> [w710 w716 w739]
          tunnel: [w710 w719 w739] -> w698
          tunnel: w696 -> [_ _ w732]
          frame "Ready", Default {
            n350 = Select(t=Hatch_Kicking_States."Stop Retaining Hatch" ("Hatch Kicking States"), s=w714, f=Hatch_Kicking_States."Ready" ("Hatch Kicking States")) -> (s? t:f=w711:T12)
          }
          frame "Stop Retaining Hatch" {
            n351 = Equal?(x=Hatch_Retainer_States."Fully Down (not retained)" ("Hatch Retainer States"), y=w716) -> (x = y?=w720:bool)
            n352 = case shown="False" w720 {
              tunnel: [Hatch_Retainer_States."Going Down" ("Hatch Retainer States") Hatch_Retainer_States."Fully Down (not retained)" ("Hatch Retainer States")] -> w719
              tunnel: [Hatch_Kicking_States."Stop Retaining Hatch" ("Hatch Kicking States") Hatch_Kicking_States."Kick Hatch" ("Hatch Kicking States")] -> w718
              frame False {
              }
              frame True {
              }
            }
          }
          frame "Kick Hatch" {
            # "if previous state\nis not the same \nas the current, we\njust entered \"kick\nhatch\" and \nshould reset our\ntimer"
            n353 = Not Equal?(x=w734, y=w732) -> (x != y?=w733:bool)
            n354 = call "Elapsed Time"("Reset"=w733) -> ("Elapsed Time (s)"=w729:dbl)  [unwired: 11 in, 7 out]
            n355 = Greater Or Equal?(x=w729, y=1.5) -> (x >= y?=w738:bool)
            n356 = Less Or Equal?(x=w729, y=0.5) -> (x <= y?=w730:bool)
            n357 = Select(t=WPI_SolenoidValue."On" ("Value"), s=w730, f=WPI_SolenoidValue."Off" ("Value")) -> (s? t:f=w731:T32)
            n358 = Select(t=Hatch_Kicking_States."Ready" ("Hatch Kicking States"), s=w738, f=Hatch_Kicking_States."Kick Hatch" ("Hatch Kicking States")) -> (s? t:f=w735:T12)
          }
        }
        n359 = Bundle By Name(cluster=w709, "Hatch Kicking States"=w704) -> (w700:T27)
        n360 = Bundle By Name(cluster=w700, "Hatch Retainer States"=w698) -> (w699:T27)
        n361 = call-poly <vilib>:"WPI_SolenoidSet.vi"("Value"=w705, "SolenoidDevRef"=w706) -> ()  [unwired: 8 in, 2 out]
      }
    }
    n362 = Unbundle By Name(w527) -> ("RetainerSolenoidDevRef"=w525:T6)
    n363 = disable-structure shown="Disabled" {
      disable-tunnel: w527 -> [w761 _]
      frame Disabled {
        n364 = Unbundle By Name(w761) -> ("Aux Button Indexes.B Button"=w768:i32)
        n365 = Unbundle By Name(w761) -> ("LifterSolenoidDevRef"=w762:T6)
        n366 = Unbundle By Name(w761) -> ("Aux Buttons"=w767:bool[])
        n367 = Index Array(array=w767, index=w768) -> (element=w764:bool)
        n368 = Select(t=WPI_SolenoidValue."On" ("Value"), s=w764, f=WPI_SolenoidValue."Off" ("Value")) -> (s? t:f=w763:T32)
        n369 = call-poly <vilib>:"WPI_SolenoidSet.vi"("Value"=w763, "SolenoidDevRef"=w762) -> ()  [unwired: 8 in, 2 out]
      }
      frame Enabled {
      }
    }
    n370 = Unbundle By Name(w527) -> ("Hatch Retainer States"=w524:T14)
    n371 = case shown="\"Going Down\"" w524 {
      tunnel: [WPI_SolenoidValue."Off" ("Value") WPI_SolenoidValue."On" ("Value") WPI_SolenoidValue."On" ("Value") WPI_SolenoidValue."Off" ("Value")] -> w523
      frame "Fully Down (not retained)", Default {
      }
      frame "Going Up" {
      }
      frame "Fully Up (retained)" {
      }
      frame "Going Down" {
      }
    }
    n372 = call-poly <vilib>:"WPI_SolenoidSet.vi"("Value"=w523, "SolenoidDevRef"=w525) -> ()  [unwired: 8 in, 2 out]
    n373 = disable-structure shown="Enabled" {
      disable-tunnel: [w596 w641] -> w539
      disable-tunnel: w528 -> [w590 w640]
      frame Disabled {
        n374 = disable-structure shown="Enabled" {
          disable-tunnel: [w600 TRUE] -> w593
          disable-tunnel: [w599 TRUE] -> w592
          disable-tunnel: w590 -> [w598 _]
          frame Disabled {
            n375 = Unbundle By Name(w598) -> ("BottomRetainerSwitchDevRef"=w602:T8)
            n376 = Unbundle By Name(w598) -> ("TopRetainerSwitchDevRef"=w604:T8)
            n377 = call <vilib>:"WPI_DigitalInputGetValue.vi"("DigitalInputDevRef"=w604) -> ("Value"=w603:bool)  [unwired: 8 in, 2 out]
            n378 = call <vilib>:"WPI_DigitalInputGetValue.vi"("DigitalInputDevRef"=w602) -> ("Value"=w601:bool)  [unwired: 8 in, 2 out]
            n379 = Not(x=w601) -> (.not. x?=w599:bool)
            n380 = Not(x=w603) -> (.not. x?=w600:bool)
          }
          frame Enabled {
            # "since we aren't using the limit\nswitches now, this acts like they're\nclicked so we don't have to rewrite\neverything"
          }
        }
        n381 = Unbundle By Name(w590) -> ("Hatch Retainer States"=w597:T14)
        n382 = Unbundle By Name(w590) -> ("HatchRetainerMotorDevRef"=w594:T1)
        n383 = Unbundle By Name(w590) -> ("Hatch Retainer Move Up/Down"=w595:bool)
        n384 = case shown="\"Going Down\"" w597 {
          tunnel: [w610 w615 w629 w634] -> w596
          tunnel: w595 -> [w613 _ w630 _]
          tunnel: w593 -> [_ w617 _ _]
          tunnel: w592 -> [_ _ _ w633]
          tunnel: w594 -> [w607 w616 w625 w632]
          tunnel: 0.2 ("Output") -> [_ w614 _ w631]
          frame "Fully Down (not retained)", Default {
            w609 = T34 0 items=["PercentOutput"=0, "Position"=1, "Velocity"=2, "Current"=3, "Follower"=5, "MotionProfile"=6, "MotionMagic"=7, "MotionProfileArc"=10, "Disabled"=15] ("Control Mode")
            n385 = call <vilib>:"CTRE_Phoenix_MotorControl_Set.vi"("Output"=0.0, "Control Mode"=w609, "PhoenixMotorControlDevRef"=w607) -> ()  [unwired: 7 in, 2 out]
            n386 = Select(t=Hatch_Retainer_States."Going Up" ("Hatch Retainer States"), s=w613, f=Hatch_Retainer_States."Fully Down (not retained)" ("Hatch Retainer States")) -> (s? t:f=w610:T14)
          }
          frame "Going Up" {
            n387 = case shown="True" w617 {
              tunnel: w616 -> [w622 _]
              tunnel: [Hatch_Retainer_States."Going Up" ("Hatch Retainer States") Hatch_Retainer_States."Fully Up (retained)" ("Hatch Retainer States")] -> w615
              tunnel: w614 -> [w619 _]
              frame False {
                w620 = T34 0 items=["PercentOutput"=0, "Position"=1, "Velocity"=2, "Current"=3, "Follower"=5, "MotionProfile"=6, "MotionMagic"=7, "MotionProfileArc"=10, "Disabled"=15] ("Control Mode")
                n388 = Negate(x=w619) -> (-x=w618:dbl)
                n389 = call <vilib>:"CTRE_Phoenix_MotorControl_Set.vi"("Output"=w618, "Control Mode"=w620, "PhoenixMotorControlDevRef"=w622) -> ()  [unwired: 7 in, 2 out]
              }
              frame True {
              }
            }
          }
          frame "Fully Up (retained)" {
            w626 = T34 0 items=["PercentOutput"=0, "Position"=1, "Velocity"=2, "Current"=3, "Follower"=5, "MotionProfile"=6, "MotionMagic"=7, "MotionProfileArc"=10, "Disabled"=15] ("Control Mode")
            n390 = call <vilib>:"CTRE_Phoenix_MotorControl_Set.vi"("Output"=0.0, "Control Mode"=w626, "PhoenixMotorControlDevRef"=w625) -> ()  [unwired: 7 in, 2 out]
            n391 = Select(t=Hatch_Retainer_States."Going Down" ("Hatch Retainer States"), s=w630, f=Hatch_Retainer_States."Fully Up (retained)" ("Hatch Retainer States")) -> (s? t:f=w629:T14)
          }
          frame "Going Down" {
            n392 = case shown="True" w633 {
              tunnel: [Hatch_Retainer_States."Going Down" ("Hatch Retainer States") Hatch_Retainer_States."Fully Down (not retained)" ("Hatch Retainer States")] -> w634
              tunnel: w632 -> [w637 _]
              tunnel: w631 -> [w635 _]
              frame False {
                w636 = T34 0 items=["PercentOutput"=0, "Position"=1, "Velocity"=2, "Current"=3, "Follower"=5, "MotionProfile"=6, "MotionMagic"=7, "MotionProfileArc"=10, "Disabled"=15] ("Control Mode")
                n393 = call <vilib>:"CTRE_Phoenix_MotorControl_Set.vi"("Output"=w635, "Control Mode"=w636, "PhoenixMotorControlDevRef"=w637) -> ()  [unwired: 7 in, 2 out]
              }
              frame True {
              }
            }
          }
        }
      }
      frame Enabled {
        n394 = disable-structure shown="Enabled" {
          disable-tunnel: [w650 TRUE] -> w644
          disable-tunnel: [w649 TRUE] -> w643
          disable-tunnel: w640 -> [w648 _]
          frame Disabled {
            n395 = Unbundle By Name(w648) -> ("BottomRetainerSwitchDevRef"=w652:T8)
            n396 = Unbundle By Name(w648) -> ("TopRetainerSwitchDevRef"=w654:T8)
            n397 = call <vilib>:"WPI_DigitalInputGetValue.vi"("DigitalInputDevRef"=w654) -> ("Value"=w653:bool)  [unwired: 8 in, 2 out]
            n398 = call <vilib>:"WPI_DigitalInputGetValue.vi"("DigitalInputDevRef"=w652) -> ("Value"=w651:bool)  [unwired: 8 in, 2 out]
            n399 = Not(x=w651) -> (.not. x?=w649:bool)
            n400 = Not(x=w653) -> (.not. x?=w650:bool)
          }
          frame Enabled {
            # "since we aren't using the limit\nswitches now, this acts like they're\nclicked so we don't have to rewrite\neverything"
          }
        }
        n401 = Unbundle By Name(w640) -> ("Hatch Retainer States"=w647:T14)
        n402 = Unbundle By Name(w640) -> ("HatchRetainerMotorDevRef"=w645:T1)
        n403 = Unbundle By Name(w640) -> ("Hatch Retainer Move Up/Down"=w646:bool)
        n404 = case shown="\"Fully Up (retained)\"" w647 {
          tunnel: [w660 Hatch_Retainer_States."Fully Up (retained)" ("Hatch Retainer States") w670 Hatch_Retainer_States."Fully Down (not retained)" ("Hatch Retainer States")] -> w641
          tunnel: w646 -> [w663 _ w671 _]
          tunnel: w644 -> [_ _ _ _]
          tunnel: w643 -> [_ _ _ _]
          tunnel: w645 -> [w657 _ w666 _]
          tunnel: 0.2 ("Output") -> [_ _ _ _]
          frame "Fully Down (not retained)", Default {
            w659 = T34 0 items=["PercentOutput"=0, "Position"=1, "Velocity"=2, "Current"=3, "Follower"=5, "MotionProfile"=6, "MotionMagic"=7, "MotionProfileArc"=10, "Disabled"=15] ("Control Mode")
            n405 = call <vilib>:"CTRE_Phoenix_MotorControl_Set.vi"("Output"=0.0, "Control Mode"=w659, "PhoenixMotorControlDevRef"=w657) -> ()  [unwired: 7 in, 2 out]
            n406 = Select(t=Hatch_Retainer_States."Going Up" ("Hatch Retainer States"), s=w663, f=Hatch_Retainer_States."Fully Down (not retained)" ("Hatch Retainer States")) -> (s? t:f=w660:T14)
          }
          frame "Going Up" {
            # "no longer need this case since \nwe switched to a pneumatic\nretainer"
          }
          frame "Fully Up (retained)" {
            w667 = T34 0 items=["PercentOutput"=0, "Position"=1, "Velocity"=2, "Current"=3, "Follower"=5, "MotionProfile"=6, "MotionMagic"=7, "MotionProfileArc"=10, "Disabled"=15] ("Control Mode")
            n407 = call <vilib>:"CTRE_Phoenix_MotorControl_Set.vi"("Output"=0.0, "Control Mode"=w667, "PhoenixMotorControlDevRef"=w666) -> ()  [unwired: 7 in, 2 out]
            n408 = Select(t=Hatch_Retainer_States."Going Down" ("Hatch Retainer States"), s=w671, f=Hatch_Retainer_States."Fully Up (retained)" ("Hatch Retainer States")) -> (s? t:f=w670:T14)
          }
          frame "Going Down" {
            # "no longer need this case since \nwe switched to a pneumatic\nretainer"
          }
        }
      }
    }
    n409 = global read "Robot Global Data.vi" "Which Robot?"() -> (w537:T30)
    n410 = global read "Robot Global Data.vi" "Which Robot?"() -> (w536:T30)
    n411 = Unbundle By Name(w528) -> ("Hatch Collector Wanted Angle"=w531:dbl)
    n412 = Unbundle By Name(w528) -> ("Hatch Collector Actual Angle"=w530:dbl)
    n413 = case shown="\"Practice Bot\"" w536 {
      tunnel: [w747 T33 {"proportional gain (Kc)"=0.0, "integral time (Ti, min)"=0.0, "derivative time (Td, min)"=0.0} ("PID gains") T33 {"proportional gain (Kc)"=0.004, "integral time (Ti, min)"=0.0, "derivative time (Td, min)"=0.0} ("PID gains")] -> w535
      frame "Competition Bot", Default {
        # "9.7% motor speed seems\nto be minimum to move"
        n414 = disable-structure shown="Enabled" {
          disable-tunnel: [T33 {"proportional gain (Kc)"=0.03, "integral time (Ti, min)"=0.003, "derivative time (Td, min)"=0.0} ("PID gains") T33 {"proportional gain (Kc)"=0.035, "integral time (Ti, min)"=0.0, "derivative time (Td, min)"=0.0} ("PID gains")] -> w747
          frame Disabled {
          }
          frame Enabled {
          }
        }
      }
      frame "Practice Bot" {
      }
      frame "Code Bot" {
        # "p = 0.008 is WAY too fast"
        # "for code bot:\nwe ended with p = 0.004,\nbut the motor has to turn\nso slowly on the code bot\nthat no PID values would\nreally work well"
      }
    }
    n415 = case shown="\"Competition Bot\", Default" w537 {
      tunnel: [cluster{"output high":dbl, "output low":dbl} {"output high"=0.2, "output low"=-0.4} ("output range") cluster{"output high":dbl, "output low":dbl} {"output high"=0.15, "output low"=-0.15} ("output range") cluster{"output high":dbl, "output low":dbl} {"output high"=0.15, "output low"=-0.15} ("output range")] -> w529
      frame "Competition Bot", Default {
      }
      frame "Practice Bot" {
      }
      frame "Code Bot" {
      }
    }
    n416 = call-poly <vilib>:"PID.vi"("output range"=w529, "PID gains"=w535, "process variable"=w530, "setpoint"=w531) -> ("output"=w559:dbl)  [unwired: 6 in, 1 out]
    n417 = Unbundle By Name(w528) -> ("HatchCollectorMotorDevRef"=w560:T1)
    n418 = call <vilib>:"WPI_MotorControlSetOutput.vi"("Output"=w559, "MotorControlDevRef"=w560) -> ()  [unwired: 7 in, 3 out]
    n419 = Bundle By Name(cluster=w528, "Hatch Retainer States"=w539) -> (w526:T27)
  }
  n420 = while {
    shift-right: [w844] -> _
    shift-left: w53 -> [w874]
    stop <- FALSE stop-if-true
    # "convert from encoder velocity to motor speed...I think"
    # "aux JS is inverted"
    n421 = Unbundle By Name(w874) -> ("DriveJoystickDevRef"=w885:T9)
    n422 = Unbundle By Name(w874) -> ("AuxJoystickDevRef"=w884:T9)
    n423 = Unbundle By Name(w874) -> ("Robot Mode"=w883:T17)
    n424 = call <vilib>:"WPI_JoystickGetValues.vi"("JoystickDevRef"=w884) -> ("Buttons"=w876:bool[], "Axes"=w877:dbl[], "JoystickDevRef"=w878:T9, "POVs"=w875:i16[])  [unwired: 6 in, 1 out]
    n425 = call <vilib>:"WPI_JoystickGetValues.vi"("JoystickDevRef"=w885) -> ("Buttons"=w880:bool[], "Axes"=w882:dbl[], "JoystickDevRef"=w881:T9, "POVs"=w879:i16[])  [unwired: 6 in, 1 out]
    n426 = Wait (ms)(milliseconds to wait=50) -> ()  [unwired: 1 out]
    n427 = case shown="\"Teleop Enabled\"" w883 {
      tunnel: w874 -> [w1064 w1074 w1075 w1076 w1086 w1087 w1088 w1098 w1099]
      tunnel: [w1064 w1065 w1075 w1077 w1086 w1087 w1088 w1089 w1099] -> w857
      tunnel: w882 -> [_ w1073 _ w1084 _ _ _ w1096 _]
      tunnel: w881 -> [_ w1072 _ w1085 _ _ _ w1097 _]
      tunnel: w880 -> [_ w1071 _ w1083 _ _ _ w1095 _]
      tunnel: w879 -> [_ w1070 _ w1082 _ _ _ w1094 _]
      tunnel: w878 -> [_ w1069 _ w1081 _ _ _ w1093 _]
      tunnel: w877 -> [_ w1068 _ w1080 _ _ _ w1092 _]
      tunnel: w876 -> [_ w1067 _ w1079 _ _ _ w1091 _]
      tunnel: w875 -> [_ w1066 _ w1078 _ _ _ w1090 _]
      frame "Autonomous Disabled", Default {
      }
      frame "Autonomous Enabled" {
        n428 = Bundle By Name(cluster=w1074, "DriveJoystickDevRef"=w1072, "Drive Axes"=w1073, "Drive Buttons"=w1071, "Drive POVs"=w1070, "AuxJoystickDevRef"=w1069, "Aux Axes"=w1068, "Aux Buttons"=w1067, "Aux POVs"=w1066) -> (w1065:T28)
      }
      frame "Teleop Disabled" {
      }
      frame "Teleop Enabled" {
        n429 = Bundle By Name(cluster=w1076, "DriveJoystickDevRef"=w1085, "Drive Axes"=w1084, "Drive Buttons"=w1083, "Drive POVs"=w1082, "AuxJoystickDevRef"=w1081, "Aux Axes"=w1080, "Aux Buttons"=w1079, "Aux POVs"=w1078) -> (w1077:T28)
      }
      frame "Disconnected" {
      }
      frame "Finish" {
      }
      frame "Test Disabled" {
      }
      frame "Test Enabled" {
        n430 = Bundle By Name(cluster=w1098, "DriveJoystickDevRef"=w1097, "Drive Axes"=w1096, "Drive Buttons"=w1095, "Drive POVs"=w1094, "AuxJoystickDevRef"=w1093, "Aux Axes"=w1092, "Aux Buttons"=w1091, "Aux POVs"=w1090) -> (w1089:T28)
      }
      frame "Emergency Stopped" {
      }
    }
    n431 = global read "Robot Global Data.vi" "Robot Mode"() -> (w859:T17)
    n432 = Bundle By Name(cluster=w857, "Robot Mode"=w859) -> (w858:T28)
    n433 = disable-structure shown="Enabled" {
      disable-tunnel: w858 -> [w990 w1034]
      disable-tunnel: w857 -> [w989 w1036]
      disable-tunnel: [_ w1021] -> w854
      frame Disabled {
        # "disabled because the RT code would override the instructions of the LT and LB code using separate bundle by names"
        # "controls both \ncylinders together"
        # "controls back cylinders only"
        # "controls front cylinders only"
        n434 = Unbundle By Name(w989) -> ("Aux Button Indexes.RT Button"=w1003:i32)
        n435 = Unbundle By Name(w989) -> ("Aux Buttons"=w1002:bool[])
        n436 = Unbundle By Name(w989) -> ("Aux Button Indexes.LT Button"=w1005:i32)
        n437 = Unbundle By Name(w989) -> ("Front Cylinders Latch"=w998:bool)
        n438 = Unbundle By Name(w989) -> ("Aux Button Indexes.LB Button"=w1020:i32)
        n439 = Unbundle By Name(w989) -> ("Aux Buttons"=w1006:bool[])
        n440 = Unbundle By Name(w989) -> ("Back Cylinders Latch"=w995:bool)
        n441 = Unbundle By Name(w989) -> ("Aux Buttons"=w1019:bool[])
        n442 = Unbundle By Name(w989) -> ("Back Cylinders Latch"=w1011:bool)
        n443 = Unbundle By Name(w989) -> ("Front Cylinders Latch"=w1014:bool)
        n444 = Index Array(array=w1002, index=w1003) -> (element=w1000:bool)
        n445 = Index Array(array=w1006, index=w1005) -> (element=w1008:bool)
        n446 = Index Array(array=w1019, index=w1020) -> (element=w1017:bool)
        n447 = feedback #10() -> (w1001:bool)  [unwired: 1 in]
        n448 = feedback-in #10(w1000) -> ()
        n449 = feedback #11() -> (w1007:bool)  [unwired: 1 in]
        n450 = feedback-in #11(w1008) -> ()
        n451 = feedback #12() -> (w1018:bool)  [unwired: 1 in]
        n452 = feedback-in #12(w1017) -> ()
        n453 = Greater?(x=w1000, y=w1001) -> (0:w994:bool)
        n454 = Greater?(x=w1008, y=w1007) -> (0:w1009:bool)
        n455 = Greater?(x=w1017, y=w1018) -> (0:w1016:bool)
        n456 = Not(x=w995) -> (.not. x?=w996:bool)
        n457 = Not(x=w998) -> (.not. x?=w999:bool)
        n458 = Not(x=w1011) -> (.not. x?=w1010:bool)
        n459 = Not(x=w1014) -> (.not. x?=w1015:bool)
        n460 = Select(t=w996, s=w994, f=w995) -> (s? t:f=w993:bool)
        n461 = Select(t=w999, s=w994, f=w998) -> (s? t:f=w997:bool)
        n462 = Select(t=w1010, s=w1009, f=w1011) -> (s? t:f=w1012:bool)
        n463 = Select(t=w1015, s=w1016, f=w1014) -> (s? t:f=w1013:bool)
        n464 = Bundle By Name(cluster=w990, "Front Cylinders Latch"=w1013) -> (w1004:T28)
        n465 = Bundle By Name(cluster=w1004, "Back Cylinders Latch"=w1012) -> (w992:T28)
        n466 = Bundle By Name(cluster=w992, "Front Cylinders Latch"=w997) -> (w991:T28)
        n467 = Bundle By Name(cluster=w991, "Back Cylinders Latch"=w993) -> (w988:T28)
      }
      frame Enabled {
        # "controls both \ncylinders together"
        # "controls back cylinders only"
        # "controls front cylinders only"
        n468 = Unbundle By Name(w1036) -> ("Aux Button Indexes.X Button"=w1040:i32)
        n469 = Unbundle By Name(w1036) -> ("Aux Buttons"=w1039:bool[])
        n470 = Unbundle By Name(w1036) -> ("Aux Button Indexes.Y Button"=w1041:i32)
        n471 = Unbundle By Name(w1036) -> ("Aux Buttons"=w1042:bool[])
        n472 = Unbundle By Name(w1036) -> ("Aux Button Indexes.A Button"=w1048:i32)
        n473 = Unbundle By Name(w1036) -> ("Aux Buttons"=w1047:bool[])
        n474 = Unbundle By Name(w1036) -> ("Front Cylinders Latch"=w1027:bool)
        n475 = Unbundle By Name(w1036) -> ("Back Cylinders Latch"=w1024:bool)
        n476 = Index Array(array=w1039, index=w1040) -> (element=w1037:bool)
        n477 = Index Array(array=w1042, index=w1041) -> (element=w1044:bool)
        n478 = Index Array(array=w1047, index=w1048) -> (element=w1045:bool)
        n479 = feedback #13() -> (w1038:bool)  [unwired: 1 in]
        n480 = feedback-in #13(w1037) -> ()
        n481 = feedback #14() -> (w1043:bool)  [unwired: 1 in]
        n482 = feedback-in #14(w1044) -> ()
        n483 = feedback #15() -> (w1046:bool)  [unwired: 1 in]
        n484 = feedback-in #15(w1045) -> ()
        n485 = Greater?(x=w1037, y=w1038) -> (0:w1031:bool)
        n486 = Greater?(x=w1044, y=w1043) -> (0:w1032:bool)
        n487 = Greater?(x=w1045, y=w1046) -> (0:w1033:bool)
        n488 = Or(x=w1033, y=w1031) -> (x .or. y?=w1030:bool)
        n489 = Or(x=w1032, y=w1031) -> (x .or. y?=w1025:bool)
        n490 = Not(x=w1027) -> (.not. x?=w1028:bool)
        n491 = Not(x=w1024) -> (.not. x?=w1026:bool)
        n492 = Select(t=w1028, s=w1030, f=w1027) -> (s? t:f=w1029:bool)
        n493 = Select(t=w1026, s=w1025, f=w1024) -> (s? t:f=w1023:bool)
        n494 = Bundle By Name(cluster=w1034, "Front Cylinders Latch"=w1029) -> (w1035:T28)
        n495 = Bundle By Name(cluster=w1035, "Back Cylinders Latch"=w1023) -> (w1022:T28)
        n496 = disable-structure shown="Disabled" {
          disable-tunnel: w1022 -> [w1053 w1055]
          disable-tunnel: [w1052 w1055] -> w1021
          frame Disabled {
            # "yaw is the angle of our robot\npitch is the angle of elevation of our robot\nroll is how much the robot is rotated about its center"
            n497 = call <vilib>:"Get_YPRHfH.vi"() -> ("YRPHfH"=w1054:T35)  [unwired: 11 in]
            n498 = Unbundle By Name(w1054) -> ("Yaw"=w1051:dbl)
            n499 = Unbundle By Name(w1054) -> ("Pitch"=w1050:dbl)
            n500 = Unbundle By Name(w1054) -> ("Roll"=w1049:dbl)
            n501 = global write "Robot Global Data.vi" "Yaw (clockwise/counter-clockwise)"(w1051) -> ()
            n502 = global write "Robot Global Data.vi" "Roll (forward/backward tipping)"(w1049) -> ()
            n503 = global write "Robot Global Data.vi" "Pitch (left/right tipping)"(w1050) -> ()
            n504 = Bundle By Name(cluster=w1053, "Yaw"=w1051, "Pitch"=w1050, "Roll"=w1049) -> (w1052:T28)
          }
          frame Enabled {
          }
        }
      }
    }
    n505 = Unbundle By Name(w854) -> ("HAB3FrontSolenoidDevRef"=w873:T6)
    n506 = Unbundle By Name(w854) -> ("HABAssisterSolenoidDevRef"=w856:T6)
    n507 = Unbundle By Name(w854) -> ("Front Cylinders Latch"=w850:bool)
    n508 = Unbundle By Name(w854) -> ("HAB3BackSolenoidDevRef"=w867:T6)
    n509 = Unbundle By Name(w854) -> ("Back Cylinders Latch"=w849:bool)
    n510 = disable-structure shown="Disabled" {
      disable-tunnel: w849 -> [w938 _]
      disable-tunnel: w854 -> [w929 _]
      disable-tunnel: [w928 w987] -> w844
      disable-tunnel: w854 -> [w927 w987]
      frame Disabled {
        w945 = T34 2 items=["PercentOutput"=0, "Position"=1, "Velocity"=2, "Current"=3, "Follower"=5, "MotionProfile"=6, "MotionMagic"=7, "MotionProfileArc"=10, "Disabled"=15] ("Control Mode")
        # "would slow down if pos. pitch, \nwhich is opposite of what we want"
        # "base spd +- PID adjustments"
        n511 = Unbundle By Name(w929) -> ("Pitch"=w951:dbl)
        n512 = global read "Robot Global Data.vi" "Which Robot?"() -> (w949:T30)
        n513 = Unbundle By Name(w929) -> ("BkSpdAdjusterMotorDevRef"=w942:T1)
        n514 = Unbundle By Name(w929) -> ("HAB Bk Spd Motor States"=w939:T13)
        n515 = global read "Robot Global Data.vi" "Which Robot?"() -> (w947:T30)
        n516 = case shown="\"Competition Bot\", Default" w947 {
          tunnel: [cluster{"output high":dbl, "output low":dbl} {"output high"=0.2, "output low"=-0.4} ("output range") cluster{"output high":dbl, "output low":dbl} {"output high"=0.15, "output low"=-0.15} ("output range") cluster{"output high":dbl, "output low":dbl} {"output high"=0.15, "output low"=-0.15} ("output range")] -> w946
          frame "Competition Bot", Default {
          }
          frame "Practice Bot" {
          }
          frame "Code Bot" {
          }
        }
        n517 = case shown="\"Code Bot\"" w949 {
          tunnel: [T33 {"proportional gain (Kc)"=0.0, "integral time (Ti, min)"=0.0, "derivative time (Td, min)"=0.0} ("PID gains") T33 {"proportional gain (Kc)"=0.0, "integral time (Ti, min)"=0.0, "derivative time (Td, min)"=0.0} ("PID gains") T33 {"proportional gain (Kc)"=0.0, "integral time (Ti, min)"=0.0, "derivative time (Td, min)"=0.0} ("PID gains")] -> w948
          tunnel: [w981 w983 w985] -> w936
          frame "Competition Bot", Default {
            w981 = 0.0  # Enc. Val at Fully Down
          }
          frame "Practice Bot" {
            w983 = 0.0  # Enc. Val at Fully Down
          }
          frame "Code Bot" {
            w985 = 0.0  # Enc. Val at Fully Down
          }
        }
        n518 = call-poly <vilib>:"PID.vi"("output range"=w946, "PID gains"=w948, "process variable"=w951, "setpoint"=0.0) -> ("output"=w944:dbl)  [unwired: 6 in, 1 out]
        n519 = global read "Robot Global Data.vi" "HAB Bk Spd Encoder Start Value"() -> (w940:dbl)
        n520 = Negate(x=w944) -> (-x=w933:dbl)
        n521 = Add(x=w933, y=0.3) -> (x+y=w934:dbl)
        n522 = call-poly <vilib>:"CTRE_Phoenix_MotorController_Get_Enhanced.vi"("PhoenixMotorControlDevRef"=w942) -> ("Quadrature Position"=w941:i32)  [unwired: 11 in, 3 out]
        n523 = Subtract(x=w941, y=w940) -> (x-y=w930:dbl)
        n524 = Greater Or Equal?(x=w930, y=w936) -> (x >= y?=w935:bool)
        n525 = Less Or Equal To 0?(x=w930) -> (x <= 0?=w931:bool)
        n526 = case shown="\"Fully Up\", Default" w939 {
          tunnel: w938 -> [w955 _ w970 _]
          tunnel: [w956 w957 w966 w972] -> w937
          tunnel: w935 -> [_ w960 _ _]
          tunnel: w934 -> [_ w959 _ _]
          tunnel: [0.0 w958 0.0 w971] -> w932
          tunnel: w931 -> [_ _ _ w973]
          frame "Fully Up", Default {
            n527 = Select(t=HAB_Bk_Spd_Motor_States."Going Down" ("HAB Bk Spd Motor States"), s=w955, f=HAB_Bk_Spd_Motor_States."Fully Up" ("HAB Bk Spd Motor States")) -> (s? t:f=w956:T13)
          }
          frame "Going Down" {
            n528 = case shown="True" w960 {
              tunnel: w959 -> [w962 _]
              tunnel: [w962 0.0] -> w958
              tunnel: [HAB_Bk_Spd_Motor_States."Going Down" ("HAB Bk Spd Motor States") HAB_Bk_Spd_Motor_States."Fully Down" ("HAB Bk Spd Motor States")] -> w957
              frame False {
              }
              frame True {
              }
            }
          }
          frame "Fully Down" {
            n529 = Not(x=w970) -> (.not. x?=w967:bool)
            n530 = Select(t=HAB_Bk_Spd_Motor_States."Going Up" ("HAB Bk Spd Motor States"), s=w967, f=HAB_Bk_Spd_Motor_States."Fully Down" ("HAB Bk Spd Motor States")) -> (s? t:f=w966:T13)
          }
          frame "Going Up" {
            n531 = case shown="True" w973 {
              tunnel: [-0.4 0.0] -> w971
              tunnel: [HAB_Bk_Spd_Motor_States."Going Up" ("HAB Bk Spd Motor States") HAB_Bk_Spd_Motor_States."Fully Up" ("HAB Bk Spd Motor States")] -> w972
              frame False {
                # "gently yeet the \nthing back up, but\nthe velocity don't\nmatter that much"
              }
              frame True {
              }
            }
          }
        }
        n532 = Bundle By Name(cluster=w927, "HAB Bk Spd Motor States"=w937) -> (w928:T28)
        n533 = call <vilib>:"CTRE_Phoenix_MotorControl_Set.vi"("Output"=w932, "Control Mode"=w945, "PhoenixMotorControlDevRef"=w942) -> ()  [unwired: 7 in, 2 out]
      }
      frame Enabled {
      }
    }
    n534 = global write "Robot Global Data.vi" "HAB Back Cylinders Extended?"(w849) -> ()
    n535 = Select(t=WPI_SolenoidValue."On" ("Value"), s=w850, f=WPI_SolenoidValue."Off" ("Value")) -> (s? t:f=w855:T32)
    n536 = global write "Robot Global Data.vi" "HAB Front Cylinders Extended?"(w850) -> ()
    n537 = call-poly <vilib>:"WPI_SolenoidSet.vi"("Value"=w855, "SolenoidDevRef"=w856) -> ()  [unwired: 8 in, 2 out]
    n538 = call-poly <vilib>:"WPI_SolenoidSet.vi"("Value"=w855, "SolenoidDevRef"=w873) -> ()  [unwired: 8 in, 2 out]
    n539 = Select(t=WPI_SolenoidValue."On" ("Value"), s=w849, f=WPI_SolenoidValue."Off" ("Value")) -> (s? t:f=w870:T32)
    n540 = call-poly <vilib>:"WPI_SolenoidSet.vi"("Value"=w870, "SolenoidDevRef"=w867) -> ()  [unwired: 8 in, 2 out]
    n541 = Unbundle By Name(w844) -> ("Aux Button Indexes.B Button"=w846:i32)
    n542 = Unbundle By Name(w844) -> ("Front HAB 3 Limit Switch"=w866:T8)
    n543 = Unbundle By Name(w844) -> ("Back HAB 3 Limit Switch"=w864:T8)
    n544 = Unbundle By Name(w844) -> ("HAB3DriveModuleMotorDevRef"=w865:T1)
    n545 = Unbundle By Name(w844) -> ("Aux Buttons"=w845:bool[])
    n546 = Unbundle By Name(w844) -> ("Aux Axes"=w862:dbl[])
    n547 = Unbundle By Name(w844) -> ("Aux Joystick Indexes.Left Y"=w863:i32)
    n548 = Unbundle By Name(w844) -> ("HAB3DriveModuleMotorDevRef"=w847:T1)
    n549 = global read "Robot Global Data.vi" "Which Robot?"() -> (w851:T30)
    n550 = disable-structure shown="Disabled" {
      disable-tunnel: w844 -> [w1056 _]
      frame Disabled {
        # "maybe use in range and coerce in future to\nprevent drivers from being able to drive\nthe module backwards?"
        # "slows down motor so\nwe don't damage the\ncylinders"
        n551 = Unbundle By Name(w1056) -> ("Aux Joystick Indexes.Right Y"=w1061:i32)
        n552 = Unbundle By Name(w1056) -> ("HAB3DriveModuleMotorDevRef"=w1063:T1)
        n553 = Unbundle By Name(w1056) -> ("Aux Axes"=w1062:dbl[])
        n554 = Index Array(array=w1062, index=w1061) -> (element=w1058:dbl)
        n555 = call "Deadband.vi"("Input"=w1058) -> ("Output"=w1059:dbl)  [unwired: 10 in]
        n556 = Multiply(x=w1059, y=0.3) -> (x*y=w1057:dbl)
        n557 = call <vilib>:"WPI_MotorControlSetOutput.vi"("Output"=w1057, "MotorControlDevRef"=w1063) -> ()  [unwired: 7 in, 3 out]
      }
      frame Enabled {
      }
    }
    n558 = call <vilib>:"WPI_DigitalInputGetValue.vi"("DigitalInputDevRef"=w864) -> ("Value"=w852:bool)  [unwired: 8 in, 2 out]
    n559 = call <vilib>:"WPI_DigitalInputGetValue.vi"("DigitalInputDevRef"=w866) -> ("Value"=w853:bool)  [unwired: 8 in, 2 out]
    n560 = Index Array(array=w862, index=w863) -> (element=w860:dbl)
    n561 = Index Array(array=w845, index=w846) -> (element=w843:bool)
    n562 = case shown="\"Practice Bot\"" w851 {
      tunnel: w853 -> [w920 w924 w926]
      tunnel: [w919 w922 w926] -> w840
      tunnel: [w918 w921 w925] -> w839
      tunnel: w852 -> [w917 w923 w925]
      frame "Competition Bot", Default {
        # "they're \ninverted\nfor some \nreason?"
        n563 = Not(x=w920) -> (.not. x?=w919:bool)
        n564 = Not(x=w917) -> (.not. x?=w918:bool)
      }
      frame "Practice Bot" {
        n565 = Not(x=w924) -> (.not. x?=w922:bool)
        n566 = Not(x=w923) -> (.not. x?=w921:bool)
      }
      frame "Code Bot" {
      }
    }
    n567 = call-poly <vilib>:"CTRE_Phoenix_MotorController_Get_Enhanced.vi"("PhoenixMotorControlDevRef"=w847) -> ("Quadrature Velocity"=w838:i32)  [unwired: 11 in, 3 out]
    n568 = Negate(x=w860) -> (-x=w848:dbl)
    n569 = disable-structure shown="Enabled" {
      disable-tunnel: w838 -> [w890 w891]
      disable-tunnel: [w889 w891] -> w837
      frame Disabled {
        n570 = Divide(x=w890, y=833) -> (x/y=w889:dbl)
      }
      frame Enabled {
      }
    }
    n571 = Or(x=w840, y=w839) -> (x .or. y?=w861:bool)
    n572 = case shown="True" w843 {
      tunnel: w865 -> [w894 w908]
      tunnel: w861 -> [w893 _]
      tunnel: w848 -> [w892 w909]
      frame False {
        n573 = case shown="False" w893 {
          tunnel: w894 -> [w896 w906]
          tunnel: w892 -> [w900 _]
          frame False {
            # "negate the negated JS so it goes forward"
            # "This is a range and coerce. :P \nSees if the joystick is going backwards.\n(If the value is negative).\nIf yes, then output is set to 0.\nIf no, then output is set from the aux\njoystick. \nWe don't want the robot to go \nbackwards off of the platform. LOL"
            # "Slows down the motor output\nso we don't damage the cylinders"
            n574 = call "Deadband.vi"("Input"=w900) -> ("Output"=w904:dbl)  [unwired: 10 in]
            n575 = In Range and Coerce(upper limit=0.0, x=w900, lower limit=-1.0) -> (In Range?=w899:bool)  [unwired: 1 out]
            n576 = Multiply(x=w904, y=0.3) -> (x*y=w895:dbl)
            n577 = Select(t=0.0, s=w899, f=w895) -> (s? t:f=w898:dbl)
            n578 = call <vilib>:"WPI_MotorControlSetOutput.vi"("Output"=w898, "MotorControlDevRef"=w896) -> ()  [unwired: 7 in, 3 out]
          }
          frame True {
            # "If either the \"Front HAB 3 Limit Switch\" or \"Front HAB 3 Limit Switch\"\nis pressed, the HAB 3 Drive Module set output will be \"0.\" \n- Preventing the DRIVER from moving too far forward into\nthe HAB 3 Platform, which can damage the cylinders.\n\nIf not, the aux joysick will control the set output.\n- Enabling the DRIVER to drive forward until the robot reaches the\nplatform"
            n579 = call <vilib>:"WPI_MotorControlSetOutput.vi"("Output"=0.0, "MotorControlDevRef"=w906) -> ()  [unwired: 7 in, 3 out]
          }
        }
      }
      frame True {
        # "if da B button is pressed, then\nit overrides the switches and\nallows the HAB Drive Mod to \ngo forward. :D!!"
        # "negate the negated JS so it goes forward"
        # "This is a range and coerce. :P \nSees if the joystick is going backwards.\n(If the value is negative).\nIf yes, then output is set to 0.\nIf no, then output is set from the aux\njoystick. \nWe don't want the robot to go \nbackwards off of the platform. LOL"
        # "Slows down the motor output\nso we don't damage the cylinders"
        n580 = call "Deadband.vi"("Input"=w909) -> ("Output"=w916:dbl)  [unwired: 10 in]
        n581 = In Range and Coerce(upper limit=0.0, x=w909, lower limit=-1.0) -> (In Range?=w912:bool)  [unwired: 1 out]
        n582 = Multiply(x=w916, y=0.3) -> (x*y=w907:dbl)
        n583 = Select(t=0.0, s=w912, f=w907) -> (s? t:f=w911:dbl)
        n584 = call <vilib>:"WPI_MotorControlSetOutput.vi"("Output"=w911, "MotorControlDevRef"=w908) -> ()  [unwired: 7 in, 3 out]
      }
    }
    n585 = global write "Robot Global Data.vi" "HAB Module Actual Velocity"(w837) -> ()
    n586 = call-poly <vilib>:"NT Write Value.vi"("Boolean"=w840, "Name"="Front HAB 3 Limit Switch") -> ()  [unwired: 9 in, 1 out]
    n587 = call-poly <vilib>:"NT Write Value.vi"("Boolean"=w839, "Name"="Back HAB 3 Limit Switch") -> ()  [unwired: 9 in, 1 out]
  }
  n588 = disable-structure shown="Enabled" {
    frame Disabled {
      # "collector \nangle \nup/down"
      # "HAB 3 drive\nmodule"
      # "RJ"
      # "LJ"
      # "angle preset hover\nfor dust pan"
      # "angle preset out/down"
      # "angle preset in/up"
      # "lift hatch"
      # "retain hatch"
      # "kick hatch"
      # "RB"
      # "RT"
      # "LB"
      # "LT"
      # "back cylinders only"
      # "both cylinders"
      # "front cylinders only"
      # "x"
      # "a"
      # "b"
      # "y"
    }
    frame Disabled {
      # "inaccurate"
      # "collector \nangle \nup/down."
      # "HAB 3 drive\nmodule."
      # "RJ"
      # "LJ"
      # "angle preset hover\nfor dust pan."
      # "angle preset out/down"
      # "angle preset in/up."
      # "lift hatch."
      # "retain hatch."
      # "kick hatch."
      # "RB"
      # "RT"
      # "LB"
      # "LT"
      # "back cylinders only."
      # "both cylinders."
      # "front cylinders only."
      # "x"
      # "a"
      # "b"
      # "y"
    }
    frame Enabled {
    }
  }
  n589 = call "Reset Drive Encoders.vi"() -> ()  [unwired: 12 in]
  "error out" <- "error in"
